vi "Complete Measurament RT (with backnoise remove).vi"() -> ()   [LabVIEW 2014]
uses:
  <vilib>/Platform/TimedLoop/XDataNode/timing_clust.ctl
  <vilib>/Platform/TimedLoop/XDataNode/nitl_modes.ctl
  <vilib>/Platform/TimedLoop/XDataNode/wakeup.ctl
  <vilib>/Analysis/3filter.llb/Filter Passband Type.ctl
  <vilib>/Analysis/Matrix/Datatypes/RealMatrix.ctl
  <vilib>/FPGAPlugInAG/sbRIO-9636/niLvFpga_Open_sbRIO-9636.vi
  <vilib>/rvi/interface/common/dynamic/niFpgaDynamicAddResources.vi
  <vilib>/FPGAPlugInAG/Dynamic/niLvFpga_Reset_Dynamic.vi
  <vilib>/Utility/error.llb/Error Cluster From Error Code.vi
  <vilib>/rvi/errors/niLvFpgaAdjustHostInterfaceError.vi
  <vilib>/Analysis/3filter.llb/Butterworth Filter (DBL).vi
  <vilib>/rvi/interface/common/niFpgaWaitOnOcc.vi
  <vilib>/FPGAPlugInAG/Dynamic/niLvFpga_Run_Dynamic.vi
  <vilib>/FPGAPlugInAG/Dynamic/niLvFpga_Abort_Dynamic.vi
  <vilib>/FPGAPlugInAG/Dynamic/niLvFpga_Close_Dynamic.vi
  <vilib>/rvi/interface/nirviOpenFPGA/nirviOpenFPGA.xnode
  FPGA Bitfiles/LaserDistanceSen_FPGATarget_N-ParametricDoub_hYmJGfBA0FM.lvbitx
  FPGA Target/Test VIs/N-Parametric Double FFT Mesurament Test SLOW (con Sottrazione Fondo).vi
  <vilib>/rvi/interface/nirviMethod/nirviMethod.xnode
  <vilib>/rvi/interface/nirviReadWriteControl/nirviReadWriteControl.xnode
  <vilib>/platform/TimedLoop/XDataNode/XDataNode.xnode
  <vilib>/rvi/interface/nirviCloseFPGA/nirviCloseFPGA.xnode
  <vilib>/FPGAPlugInAG/Dynamic/niLvFpga_ConfigureFifo_Dynamic.vi
  <vilib>/rvi/errors/niLvFpgaMergeErrorWithErrorCode.vi
  <vilib>/FPGAPlugInAG/Dynamic/niLvFpga_StartFifo_Dynamic.vi
  <vilib>/rvi/interface/Simulation/niFpgaSimulationCallBeginRW.vi
  <vilib>/FPGAPlugInAG/Dynamic/niLvFpga_ReadFifo_Dynamic.vi
  <vilib>/Platform/TimedLoop/XDataNode/XDNodeRunTimeDep.lvlib
  NiFpgaLv.dll
  <vilib>/Analysis/NI_AALBase.lvlib
  <vilib>/Analysis/Matrix/NI_Matrix.lvlib
panel:
  out "Array":i32[](array[numeric])
  out "mean distance size":i32
  in  "n-bit (2^nbit medie)":i32=8
  in  "Savitzy golay: polynomial order":i32=3
  in  "Savitzy golay: side points":i32=6
  in  "LowPass Filter: Low cutoff frequency":dbl=1000000.0 format="%#_13g"
  in  "PolyFitting: Poly Grade":dbl=5.0
  in  "SubtractionType":T1(ring)=enum."LowPass"
  out "Fondo Signal":dbl[](graph)
  out "Distance ONLINE":dbl[](graph)
  in  "Low cutoff freq":dbl=200000.0 format="%#_13g"
  in  "Tri Low pass filter":bool
  in  "3 point interpolation algorithm":bool
  in  "Mov mean":bool
  out "moving mean speed":dbl format="%0.7f"
  out "moving standard deviation rel speed":dbl format="%0.7f"
  in  "#movesignal 2":i32=100
  out "moving freq mean":dbl
  in  "Tab Control":enum32{"5 bin", "5 bin mean", "Distance "}(tab)=enum."Distance "
  out "5 bin FALL":T2(graph) caption="5 freq fall"
  out "5 bin RISE":T2(graph)
  out "5 bin mean/std FALL":T3(graph)
  in  "#meanBin":i32=100
  out "5 bin mean/std RISE":T3(graph)
  out "Distance and error":T2(graph)
  out "Speed and error":T2(graph)
  in  "Lin Mes":bool
  in  "step (m)":dbl=0.0001
  out "Max peak-peak error (m)":dbl
  out "Mean error (m)":dbl
  in  "Plot":bool
  in  "Sample /Modulation Frequency":enum32{"40MHz/32KHz", "30MHz/24Khz"}(radio)=enum."30MHz/24Khz"
  in  "#movesignal":i32=100
  out "moving standard deviation rel":dbl format="%0.7f"
  out "moving mean":dbl format="%0.7f"
  out "StdDev Rel 1":dbl
  out "StdDev Rel 2":dbl
  out "Warning":bool
  out "Velocity (m/s)":dbl
  out "Distance (m)":dbl
  out "Mean Frequency":dbl
  out "Rise array size":i32
  out "Fall array size":i32
  out "Mean Frequency Rising (Hz)":dbl
  out "Mean Frequency Falling (Hz)":dbl
  in  "tieni premuto per":i32=100
  in  "Triangular Multiply Factor":dbl[](array[numeric])=[1.0, 0.8, 0.95, 0.85, 0.9]
  out "RISING Second Edge N-FFT":dbl[](graph)
  in  "Enable triangular scaling":bool=TRUE
  in  "Triangolo dritto?":bool
  out "FALLING First Edge N-FFT":dbl[](graph)
  in  "#Signals":u32(slide)=5 scale=1.0..5.0
  in  "stop":bool
  in  "Initial Latency points":u32(slide)=260 scale=0.0..1249.0
  out "Elements Remaining FFT":u32
  out "Elements Remaining Signal":u32
  out "N-Signals":dbl[](graph)
  in  "Snapshot":bool
  in  "Windowing":T4(ring)=enum."Hanning"
  in  "first bin":i32=5
  in  "last bin":i32=255
  in  "lower limit 2":u32(slide)=738 scale=625.0..738.0
  in  "lower limit 1":u32(slide)=113 scale=0.0..113.0
  # "SOTTRAZIONE FONDO"
  # "OFFLINE parameters"
  # "200k/400k"
  # "Max Detection FFT bin range"
  # "WARNING:\nOnce pressed wait untill the end of operation"
  # "Distance"
  # "Mean"
  # "Velocity"
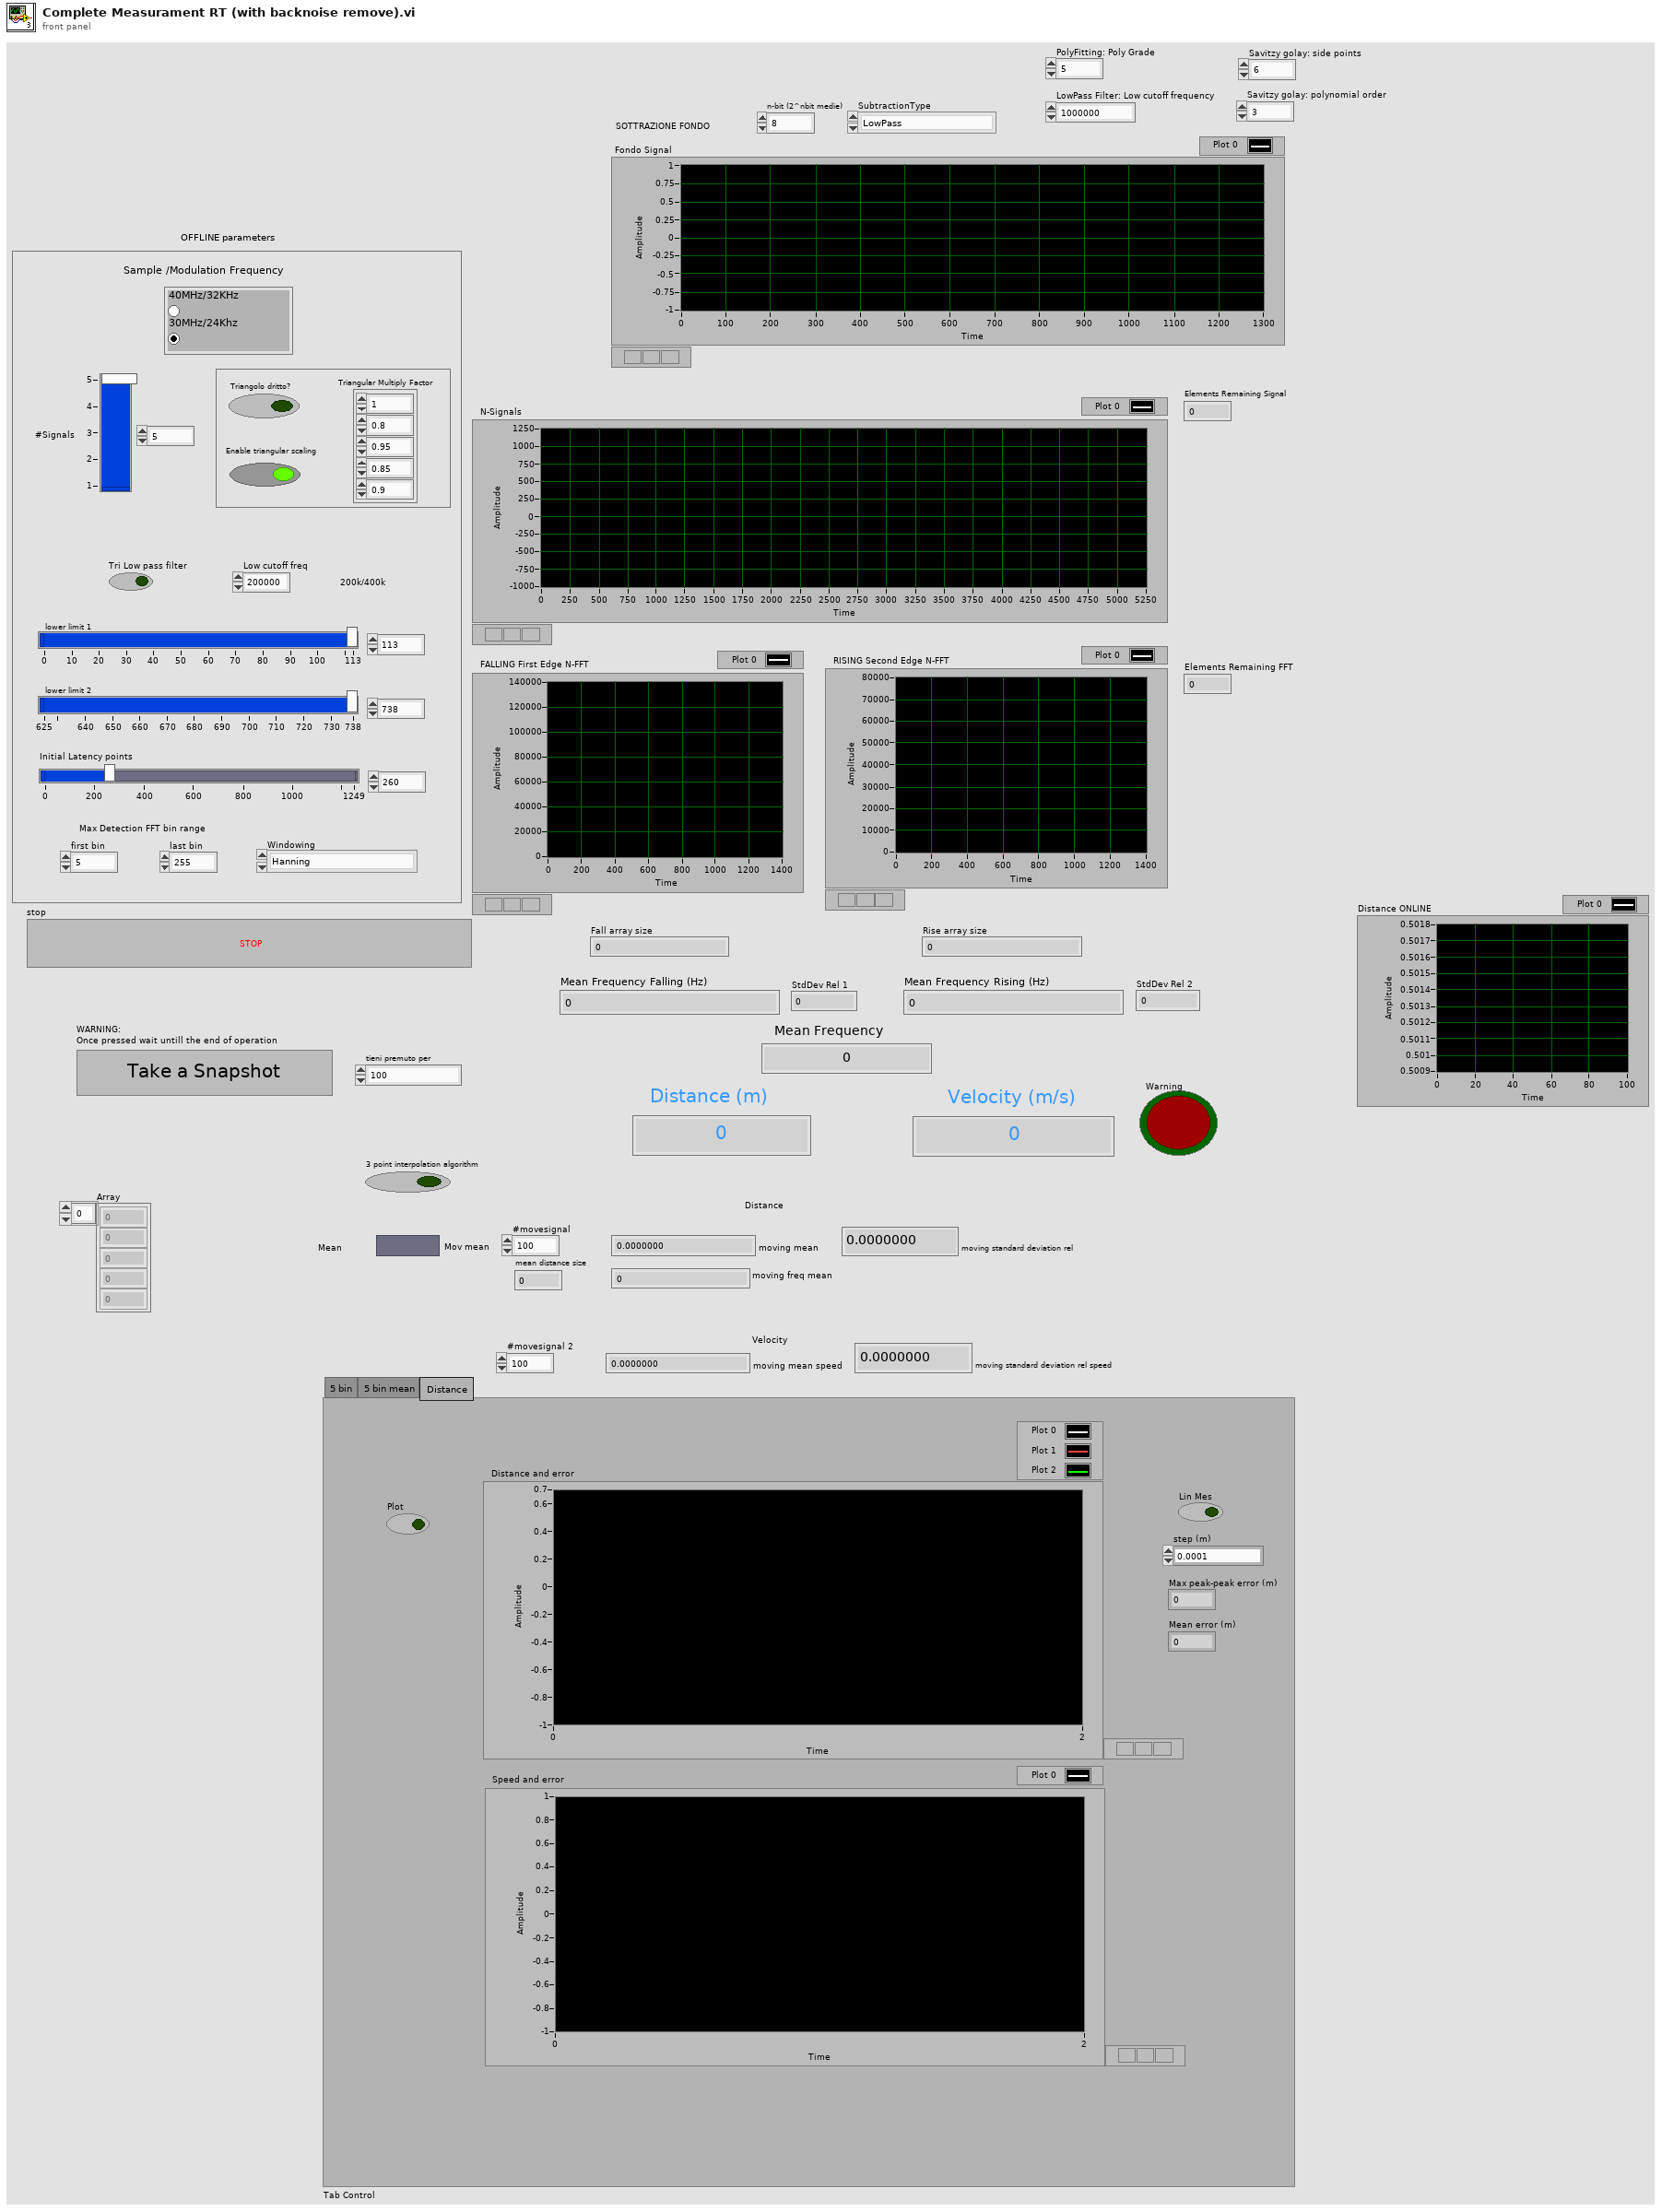
[diagram p1: front panel]
types:
  T1 = enum16{"NoSubtract", "StartingCurve", "LowPass", "PolyFitting", "SavGolay"}
  T2 = cluster{"[0]":dbl, "[1]":dbl, "[2]":dbl, "[3]":dbl, "[4]":dbl, "[5]":dbl, "[6]":dbl, "[7]":dbl, "[8]":dbl}
  T3 = cluster{"Array[0]":dbl, "Array[1]":dbl, "Array[2]":dbl, "Array[3]":dbl, "Array[4]":dbl, "Array[5]":dbl, "Array[6]":dbl, "Array[7]":dbl, "Array[8]":dbl}
  T4 = enum16{"None", "Hanning", "Hamming", "Blackman", "Blackman-Harris"}
  T5 = typedef "NI_AALBase.lvlib/Filter Passband Type.ctl" = enum32{"Lowpass", "Highpass", "Bandpass", "Bandstop"}
  T6 = typedef "XDNodeRunTimeDep.lvlib/timing_clust.ctl" = cluster{"Expected End [f-1]":u64, "Actual End [f-1]":u64, "Finished Late? [f-1]":bool, "Expected End [i-1]":u64, "Actual End [i-1]":u64, "Finished Late? [i-1]":bool, "Expected Start [i]":u64, "Actual Start [i]":u64, "Expected Start [f]":u64, "Actual Start [f]":u64, "Source Name":string, "Structure Name":string, "Period":i64, "Deadline":i64, "Offset":i64, "Start":i64, "Priority":i32, "Timeout":i32, "Mode":T7, "Wakeup Reason":T8, "Error":errorcluster, "Source Type":string, "Secondary Source Type":string, "Global End Time":u64, "Global Start Time":u64, "Frame Duration":u64, "Iteration Duration":u64, "Assigned CPU":i32, "I/O Scan Engine Mode":u32}
  T7 = typedef "XDNodeRunTimeDep.lvlib/nitl_modes.ctl" = enum32{"No Change", "Process missed periods, maintain original phase", "Discard missed periods, maintain original phase", "Process missed periods, ignore original phase", "Discard missed periods, ignore original phase"}
  T8 = typedef "XDNodeRunTimeDep.lvlib/wakeup.ctl" = enum32{"Normal", "Aborted", "Asynchronous wakeup", "Timing source error", "Timed loop error", "Timeout"}
  T9 = typedef "NI_Matrix.lvlib/RealMatrix.ctl" = dbl[][]
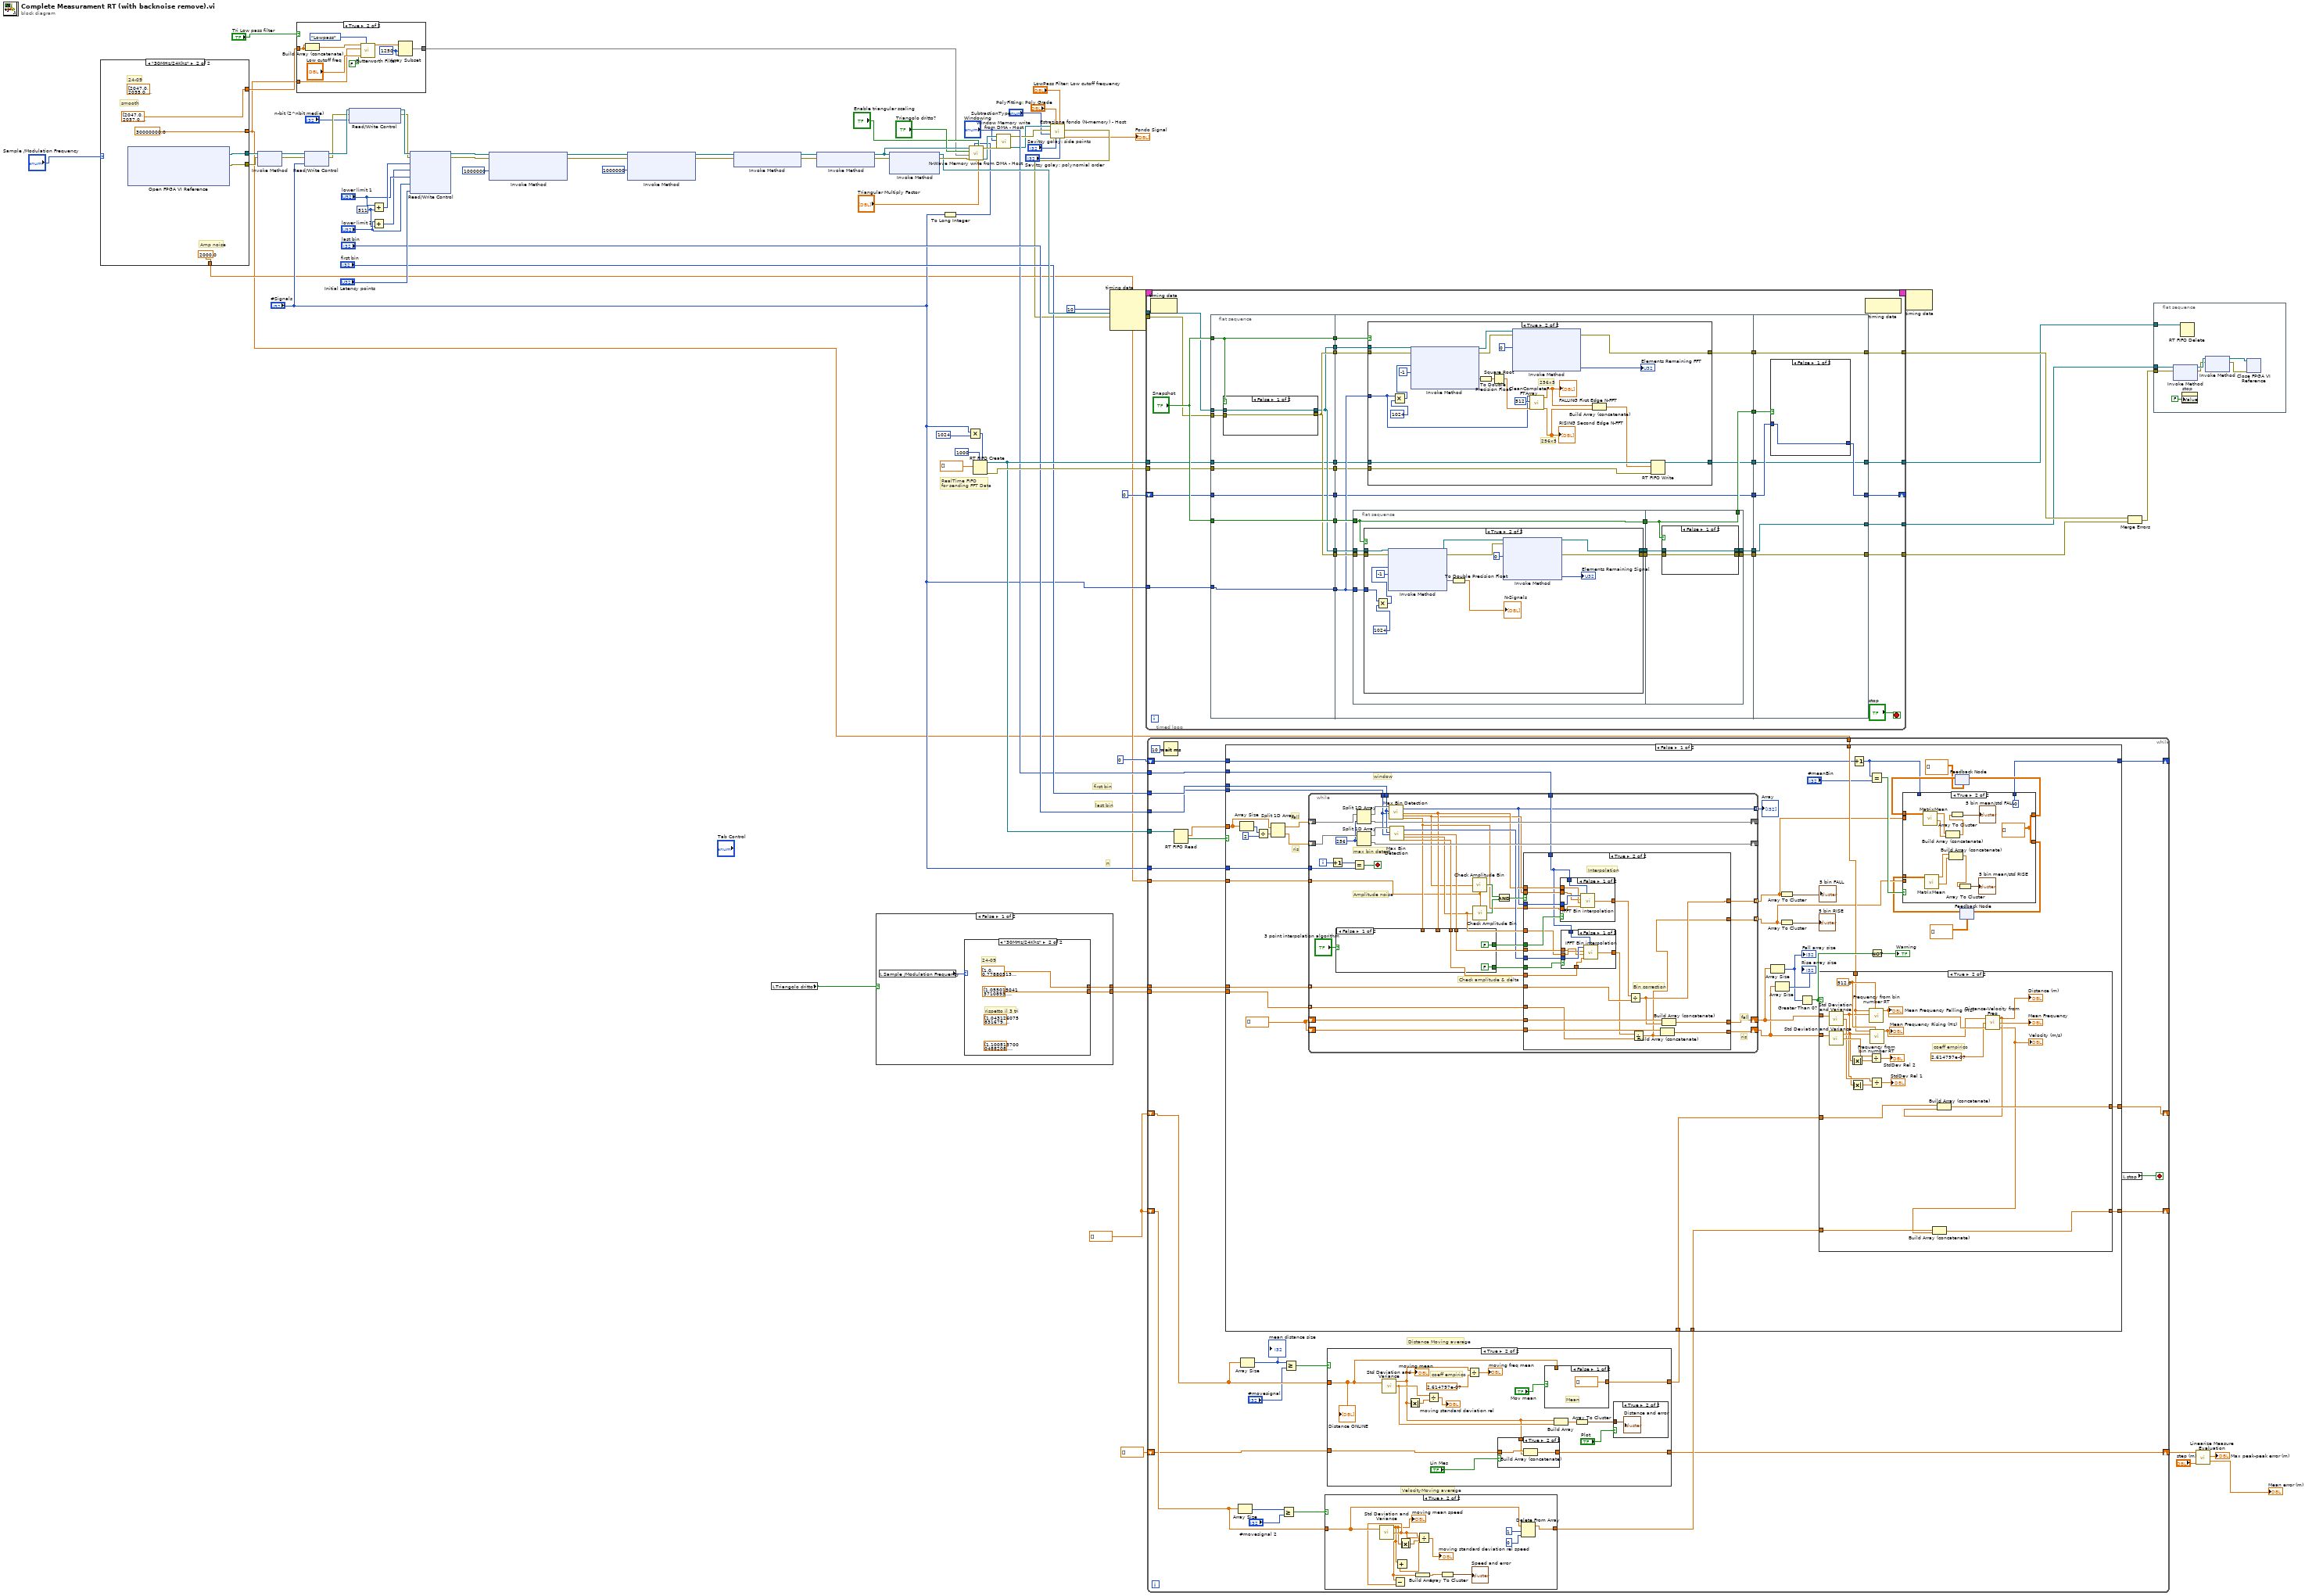
[diagram p0: block diagram]
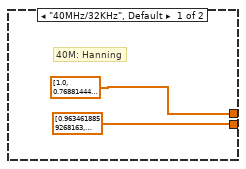
[diagram p3: hidden frame]
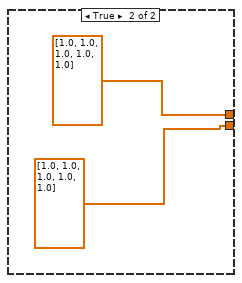
[diagram p4: hidden frame]
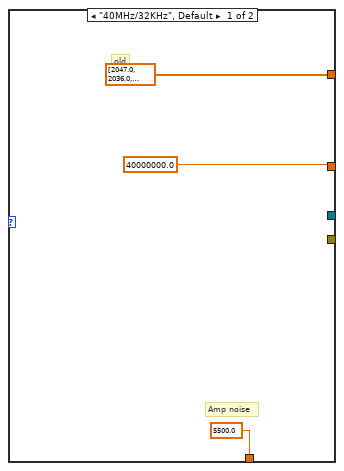
[diagram p5: hidden frame]
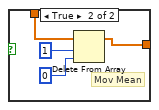
[diagram p10: hidden frame]
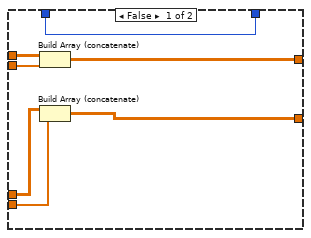
[diagram p11: hidden frame]
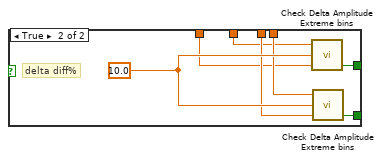
[diagram p13: hidden frame]
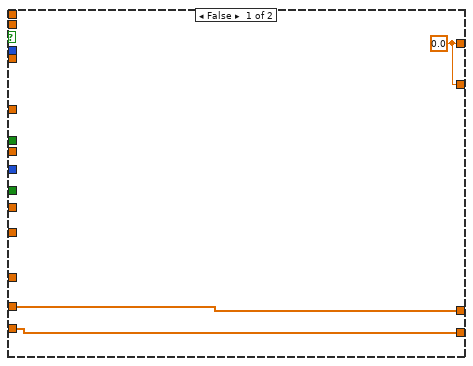
[diagram p14: hidden frame]
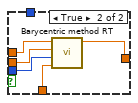
[diagram p15: hidden frame]
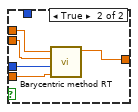
[diagram p16: hidden frame]
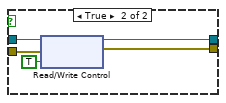
[diagram p18: hidden frame]
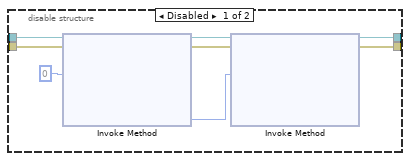
[diagram p20: hidden frame]
diagram:
  w25 = dbl[] [] ("appended array")
  w75 = u32 511 ("y")
  # "n"
  # "last bin"
  # "first bin"
  # "RealTime FIFO \nfor sending FFT Data"
  n1 = case shown="\"30MHz/24Khz\"" "Sample /Modulation Frequency" {
    tunnel: [_ w87] -> w50
    tunnel: [_ w86] -> w49
    tunnel: [40000000.0 30000000.0] -> w21
    tunnel: [5500.0 ("Threshold Amp") 2000.0 ("Threshold Amp")] -> w26
    tunnel: [dbl[] [2047.0, 2036.0, 2024.0, 2013.0, 2002.0, 1990.0, 1979.0, 1968.0, 1956.0, 1945.0, 1934.0, 1923.0, 1912.0, 1900.0, 1889.0, 1878.0, 1867.0, 1856.0, 1845.0, 1833.0, 1822.0, 1811.0, 1800.0, 1789.0, 1778.0, 1767.0, 1756.0, 1745.0, 1734.0, 1723.0, 1712.0, 1702.0, 1691.0, 1680.0, 1669.0, 1658.0, 1647.0, 1636.0, 1626.0, 1615.0, 1604.0, 1593.0, 1583.0, 1572.0, 1561.0, 1550.0, 1540.0, 1529.0, 1518.0, 1508.0, 1497.0, 1487.0, 1476.0, 1465.0, 1455.0, 1444.0, 1434.0, 1423.0, 1413.0, 1402.0, 1392.0, 1381.0, 1371.0, 1360.0, 1350.0, 1340.0, 1329.0, 1319.0, 1309.0, 1298.0, 1288.0, 1278.0, 1267.0, 1257.0, 1247.0, 1237.0, 1226.0, 1216.0, 1206.0, 1196.0, 1186.0, 1176.0, 1165.0, 1155.0, 1145.0, 1135.0, 1125.0, 1115.0, 1105.0, 1095.0, 1085.0, 1075.0, 1065.0, 1055.0, 1045.0, 1035.0, 1025.0, 1015.0, 1006.0, 996.0, 986.0, 976.0, 966.0, 956.0, 947.0, 937.0, 927.0, 917.0, 908.0, 898.0, 888.0, 879.0, 869.0, 859.0, 850.0, 837.0, 826.0, 816.0, 804.0, 796.0, 788.0, 778.0, 769.0, 758.0, 750.0, 743.0, 733.0, 724.0, 717.0, 709.0, 701.0, 693.0, 686.0, 677.0, 669.0, 661.0, 653.0, 645.0, 638.0, 630.0, 622.0, 615.0, 607.0, 599.0, 592.0, 583.0, 576.0, 569.0, 561.0, 554.0, 547.0, 539.0, 532.0, 525.0, 518.0, 509.0, 501.0, 492.0, 486.0, 478.0, 471.0, 463.0, 456.0, 450.0, 442.0, 435.0, 429.0, 421.0, 415.0, 408.0, 401.0, 394.0, 388.0, 381.0, 375.0, 368.0, 361.0, 355.0, 349.0, 342.0, 336.0, 330.0, 323.0, 317.0, 311.0, 304.0, 298.0, 292.0, 286.0, 279.0, 273.0, 267.0, 261.0, 255.0, 249.0, 242.0, 236.0, 230.0, 224.0, 218.0, 212.0, 206.0, 200.0, 194.0, 187.0, 181.0, 175.0, 169.0, 163.0, 157.0, 150.0, 144.0, 138.0, 132.0, 125.0, 119.0, 113.0, 107.0, 101.0, 95.0, 88.0, 82.0, 77.0, 71.0, 65.0, 59.0, 53.0, 47.0, 41.0, 35.0, 29.0, 23.0, 18.0, 11.0, 6.0, 0.0, -6.0, -12.0, -18.0, -23.0, -29.0, -35.0, -41.0, -47.0, -52.0, -58.0, -64.0, -69.0, -75.0, -81.0, -87.0, -92.0, -98.0, -104.0, -109.0, -115.0, -121.0, -126.0, -132.0, -138.0, -144.0, -149.0, -155.0, -161.0, -166.0, -172.0, -177.0, -183.0, -189.0, -194.0, -200.0, -205.0, -211.0, -216.0, -222.0, -227.0, -233.0, -238.0, -244.0, -249.0, -255.0, -260.0, -266.0, -271.0, -277.0, -283.0, -288.0, -294.0, -299.0, -304.0, -310.0, -315.0, -321.0, -326.0, -331.0, -337.0, -342.0, -348.0, -353.0, -358.0, -364.0, -369.0, -375.0, -380.0, -385.0, -391.0, -396.0, -402.0, -407.0, -413.0, -418.0, -423.0, -429.0, -434.0, -439.0, -445.0, -450.0, -456.0, -461.0, -466.0, -472.0, -477.0, -483.0, -488.0, -493.0, -499.0, -504.0, -510.0, -515.0, -520.0, -526.0, -531.0, -537.0, -542.0, -548.0, -553.0, -558.0, -564.0, -569.0, -574.0, -580.0, -585.0, -590.0, -596.0, -601.0, -606.0, -612.0, -617.0, -622.0, -628.0, -633.0, -638.0, -644.0, -649.0, -654.0, -660.0, -665.0, -670.0, -676.0, -681.0, -686.0, -692.0, -697.0, -702.0, -708.0, -713.0, -718.0, -723.0, -729.0, -734.0, -739.0, -744.0, -750.0, -755.0, -760.0, -765.0, -771.0, -776.0, -781.0, -786.0, -792.0, -797.0, -802.0, -807.0, -812.0, -818.0, -823.0, -828.0, -833.0, -839.0, -844.0, -849.0, -854.0, -859.0, -865.0, -870.0, -875.0, -880.0, -885.0, -891.0, -896.0, -901.0, -906.0, -911.0, -916.0, -922.0, -927.0, -932.0, -937.0, -943.0, -948.0, -953.0, -958.0, -963.0, -969.0, -974.0, -979.0, -984.0, -989.0, -995.0, -1000.0, -1005.0, -1010.0, -1015.0, -1021.0, -1026.0, -1031.0, -1036.0, -1041.0, -1047.0, -1052.0, -1057.0, -1062.0, -1067.0, -1073.0, -1078.0, -1083.0, -1088.0, -1093.0, -1099.0, -1104.0, -1109.0, -1114.0, -1119.0, -1124.0, -1130.0, -1135.0, -1140.0, -1145.0, -1150.0, -1156.0, -1161.0, -1166.0, -1171.0, -1176.0, -1182.0, -1187.0, -1192.0, -1197.0, -1202.0, -1207.0, -1213.0, -1218.0, -1223.0, -1228.0, -1233.0, -1238.0, -1244.0, -1249.0, -1254.0, -1259.0, -1264.0, -1269.0, -1275.0, -1280.0, -1285.0, -1290.0, -1295.0, -1300.0, -1305.0, -1311.0, -1316.0, -1321.0, -1326.0, -1331.0, -1336.0, -1342.0, -1347.0, -1352.0, -1357.0, -1362.0, -1367.0, -1372.0, -1378.0, -1383.0, -1388.0, -1393.0, -1398.0, -1403.0, -1408.0, -1414.0, -1419.0, -1424.0, -1429.0, -1434.0, -1439.0, -1444.0, -1450.0, -1455.0, -1460.0, -1465.0, -1470.0, -1475.0, -1480.0, -1486.0, -1491.0, -1496.0, -1501.0, -1506.0, -1511.0, -1516.0, -1522.0, -1527.0, -1532.0, -1537.0, -1542.0, -1547.0, -1552.0, -1558.0, -1563.0, -1568.0, -1573.0, -1578.0, -1583.0, -1588.0, -1593.0, -1599.0, -1604.0, -1609.0, -1614.0, -1619.0, -1624.0, -1629.0, -1634.0, -1640.0, -1645.0, -1650.0, -1655.0, -1660.0, -1665.0, -1670.0, -1675.0, -1681.0, -1686.0, -1691.0, -1696.0, -1701.0, -1706.0, -1711.0, -1716.0, -1722.0, -1727.0, -1732.0, -1737.0, -1742.0, -1747.0, -1752.0, -1757.0, -1762.0, -1768.0, -1773.0, -1778.0, -1783.0, -1788.0, -1793.0, -1798.0, -1803.0, -1808.0, -1814.0, -1819.0, -1824.0, -1829.0, -1834.0, -1839.0, -1844.0, -1849.0, -1854.0, -1859.0, -1865.0, -1870.0, -1875.0, -1880.0, -1885.0, -1890.0, -1895.0, -1900.0, -1905.0, -1911.0, -1916.0, -1921.0, -1926.0, -1931.0, -1936.0, -1941.0, -1946.0, -1951.0, -1956.0, -1961.0, -1967.0, -1972.0, -1977.0, -1982.0, -1987.0, -1992.0, -1997.0, -2002.0, -2007.0, -2012.0, -2017.0, -2023.0, -2028.0, -2033.0, -2038.0, -2043.0, -2048.0, -2047.0, -2034.0, -2021.0, -2009.0, -1996.0, -1983.0, -1970.0, -1957.0, -1945.0, -1932.0, -1919.0, -1907.0, -1894.0, -1881.0, -1869.0, -1856.0, -1844.0, -1831.0, -1819.0, -1806.0, -1794.0, -1781.0, -1769.0, -1757.0, -1744.0, -1732.0, -1719.0, -1707.0, -1695.0, -1682.0, -1670.0, -1658.0, -1646.0, -1634.0, -1621.0, -1609.0, -1597.0, -1585.0, -1573.0, -1561.0, -1549.0, -1537.0, -1525.0, -1513.0, -1501.0, -1489.0, -1477.0, -1465.0, -1453.0, -1441.0, -1429.0, -1417.0, -1405.0, -1394.0, -1382.0, -1370.0, -1358.0, -1347.0, -1335.0, -1323.0, -1312.0, -1300.0, -1288.0, -1277.0, -1265.0, -1254.0, -1242.0, -1231.0, -1219.0, -1208.0, -1196.0, -1185.0, -1173.0, -1162.0, -1150.0, -1139.0, -1128.0, -1116.0, -1105.0, -1094.0, -1083.0, -1071.0, -1060.0, -1049.0, -1038.0, -1027.0, -1015.0, -1004.0, -993.0, -982.0, -971.0, -960.0, -949.0, -938.0, -927.0, -916.0, -905.0, -894.0, -883.0, -873.0, -862.0, -851.0, -840.0, -829.0, -819.0, -808.0, -797.0, -786.0, -776.0, -765.0, -754.0, -744.0, -733.0, -722.0, -712.0, -697.0, -685.0, -674.0, -661.0, -652.0, -643.0, -632.0, -622.0, -610.0, -602.0, -594.0, -583.0, -574.0, -566.0, -558.0, -550.0, -542.0, -534.0, -525.0, -516.0, -507.0, -499.0, -491.0, -483.0, -475.0, -467.0, -459.0, -451.0, -443.0, -435.0, -426.0, -419.0, -411.0, -404.0, -396.0, -388.0, -381.0, -373.0, -366.0, -359.0, -349.0, -341.0, -331.0, -325.0, -317.0, -309.0, -301.0, -295.0, -288.0, -280.0, -273.0, -266.0, -259.0, -252.0, -246.0, -239.0, -231.0, -225.0, -219.0, -212.0, -205.0, -199.0, -192.0, -186.0, -180.0, -173.0, -167.0, -161.0, -155.0, -148.0, -142.0, -136.0, -130.0, -124.0, -118.0, -112.0, -106.0, -100.0, -94.0, -88.0, -82.0, -76.0, -70.0, -64.0, -58.0, -52.0, -46.0, -40.0, -34.0, -28.0, -21.0, -15.0, -9.0, -3.0, 2.0, 9.0, 15.0, 21.0, 27.0, 33.0, 39.0, 45.0, 51.0, 57.0, 63.0, 69.0, 75.0, 81.0, 86.0, 92.0, 98.0, 103.0, 110.0, 116.0, 121.0, 127.0, 133.0, 138.0, 144.0, 149.0, 155.0, 161.0, 166.0, 172.0, 177.0, 183.0, 189.0, 194.0, 200.0, 205.0, 211.0, 216.0, 221.0, 227.0, 232.0, 238.0, 243.0, 249.0, 254.0, 259.0, 265.0, 270.0, 276.0, 281.0, 286.0, 292.0, 297.0, 303.0, 308.0, 314.0, 319.0, 324.0, 329.0, 335.0, 340.0, 345.0, 351.0, 356.0, 361.0, 366.0, 371.0, 377.0, 382.0, 387.0, 392.0, 397.0, 403.0, 408.0, 413.0, 418.0, 423.0, 429.0, 434.0, 439.0, 444.0, 449.0, 454.0, 459.0, 464.0, 469.0, 474.0, 479.0, 484.0, 489.0, 494.0, 499.0, 504.0, 509.0, 514.0, 520.0, 525.0, 530.0, 535.0, 540.0, 545.0, 550.0, 555.0, 560.0, 565.0, 570.0, 575.0, 580.0, 585.0, 590.0, 595.0, 600.0, 605.0, 610.0, 615.0, 620.0, 625.0, 630.0, 636.0, 641.0, 646.0, 651.0, 656.0, 661.0, 666.0, 671.0, 676.0, 681.0, 686.0, 691.0, 696.0, 701.0, 706.0, 711.0, 716.0, 721.0, 726.0, 731.0, 736.0, 741.0, 746.0, 751.0, 756.0, 761.0, 765.0, 770.0, 775.0, 780.0, 785.0, 790.0, 795.0, 800.0, 805.0, 810.0, 815.0, 820.0, 825.0, 829.0, 834.0, 839.0, 844.0, 849.0, 854.0, 859.0, 864.0, 868.0, 873.0, 878.0, 883.0, 888.0, 893.0, 897.0, 902.0, 907.0, 912.0, 917.0, 921.0, 926.0, 931.0, 936.0, 941.0, 945.0, 950.0, 955.0, 960.0, 965.0, 969.0, 974.0, 979.0, 984.0, 988.0, 993.0, 998.0, 1003.0, 1007.0, 1012.0, 1017.0, 1022.0, 1027.0, 1031.0, 1036.0, 1041.0, 1046.0, 1051.0, 1055.0, 1060.0, 1065.0, 1070.0, 1075.0, 1079.0, 1084.0, 1089.0, 1094.0, 1098.0, 1103.0, 1108.0, 1113.0, 1118.0, 1122.0, 1127.0, 1132.0, 1137.0, 1141.0, 1146.0, 1151.0, 1156.0, 1161.0, 1165.0, 1170.0, 1175.0, 1180.0, 1184.0, 1189.0, 1194.0, 1199.0, 1204.0, 1208.0, 1213.0, 1218.0, 1223.0, 1227.0, 1232.0, 1237.0, 1242.0, 1246.0, 1251.0, 1256.0, 1261.0, 1265.0, 1270.0, 1275.0, 1280.0, 1284.0, 1289.0, 1294.0, 1299.0, 1303.0, 1308.0, 1313.0, 1318.0, 1322.0, 1327.0, 1332.0, 1336.0, 1341.0, 1346.0, 1351.0, 1355.0, 1360.0, 1365.0, 1370.0, 1374.0, 1379.0, 1384.0, 1388.0, 1393.0, 1398.0, 1403.0, 1407.0, 1412.0, 1417.0, 1421.0, 1426.0, 1431.0, 1436.0, 1440.0, 1445.0, 1450.0, 1454.0, 1459.0, 1464.0, 1469.0, 1473.0, 1478.0, 1483.0, 1487.0, 1492.0, 1497.0, 1502.0, 1506.0, 1511.0, 1516.0, 1520.0, 1525.0, 1530.0, 1535.0, 1539.0, 1544.0, 1549.0, 1553.0, 1558.0, 1563.0, 1567.0, 1572.0, 1577.0, 1582.0, 1586.0, 1591.0, 1596.0, 1600.0, 1605.0, 1610.0, 1614.0, 1619.0, 1624.0, 1628.0, 1633.0, 1638.0, 1643.0, 1647.0, 1652.0, 1657.0, 1661.0, 1666.0, 1671.0, 1675.0, 1680.0, 1685.0, 1689.0, 1694.0, 1699.0, 1703.0, 1708.0, 1713.0, 1717.0, 1722.0, 1727.0, 1731.0, 1736.0, 1741.0, 1746.0, 1750.0, 1755.0, 1760.0, 1764.0, 1769.0, 1774.0, 1778.0, 1783.0, 1788.0, 1792.0, 1797.0, 1802.0, 1806.0, 1811.0, 1816.0, 1820.0, 1825.0, 1830.0, 1834.0, 1839.0, 1844.0, 1848.0, 1853.0, 1858.0, 1862.0, 1867.0, 1871.0, 1876.0, 1881.0, 1885.0, 1890.0, 1895.0, 1899.0, 1904.0, 1909.0, 1913.0, 1918.0, 1923.0, 1927.0, 1932.0, 1937.0, 1941.0, 1946.0, 1951.0, 1955.0, 1960.0, 1965.0, 1969.0, 1974.0, 1978.0, 1983.0, 1988.0, 1992.0, 1997.0, 2002.0, 2006.0, 2011.0, 2016.0, 2020.0, 2025.0, 2029.0, 2034.0, 2039.0, 2043.0, 2048.0] ("Complete SkewTri") dbl[] [2047.0, 2037.0, 2027.0, 2018.0, 2008.0, 1998.0, 1989.0, 1979.0, 1969.0, 1960.0, 1950.0, 1940.0, 1931.0, 1921.0, 1911.0, 1902.0, 1892.0, 1882.0, 1873.0, 1863.0, 1854.0, 1844.0, 1835.0, 1825.0, 1816.0, 1806.0, 1797.0, 1787.0, 1778.0, 1768.0, 1759.0, 1749.0, 1740.0, 1730.0, 1721.0, 1711.0, 1702.0, 1693.0, 1683.0, 1674.0, 1665.0, 1655.0, 1646.0, 1637.0, 1627.0, 1618.0, 1609.0, 1599.0, 1590.0, 1581.0, 1572.0, 1562.0, 1553.0, 1544.0, 1535.0, 1525.0, 1516.0, 1507.0, 1498.0, 1489.0, 1479.0, 1470.0, 1461.0, 1452.0, 1443.0, 1434.0, 1425.0, 1416.0, 1407.0, 1398.0, 1388.0, 1379.0, 1370.0, 1361.0, 1352.0, 1343.0, 1334.0, 1325.0, 1316.0, 1307.0, 1299.0, 1290.0, 1281.0, 1272.0, 1263.0, 1254.0, 1245.0, 1236.0, 1227.0, 1218.0, 1210.0, 1201.0, 1192.0, 1183.0, 1174.0, 1166.0, 1157.0, 1148.0, 1139.0, 1130.0, 1122.0, 1113.0, 1104.0, 1096.0, 1087.0, 1078.0, 1069.0, 1061.0, 1052.0, 1043.0, 1035.0, 1026.0, 1018.0, 1009.0, 1000.0, 992.0, 983.0, 975.0, 966.0, 958.0, 950.0, 941.0, 933.0, 925.0, 917.0, 908.0, 900.0, 892.0, 884.0, 876.0, 868.0, 860.0, 852.0, 844.0, 837.0, 829.0, 821.0, 813.0, 805.0, 798.0, 790.0, 782.0, 775.0, 767.0, 760.0, 752.0, 745.0, 737.0, 730.0, 722.0, 715.0, 707.0, 700.0, 693.0, 685.0, 678.0, 671.0, 664.0, 656.0, 649.0, 642.0, 635.0, 628.0, 621.0, 613.0, 606.0, 599.0, 592.0, 585.0, 578.0, 571.0, 564.0, 557.0, 550.0, 543.0, 537.0, 530.0, 523.0, 516.0, 509.0, 502.0, 495.0, 489.0, 482.0, 475.0, 468.0, 462.0, 455.0, 448.0, 442.0, 435.0, 428.0, 422.0, 415.0, 408.0, 402.0, 395.0, 389.0, 382.0, 375.0, 369.0, 362.0, 356.0, 349.0, 343.0, 336.0, 330.0, 324.0, 317.0, 311.0, 304.0, 298.0, 291.0, 285.0, 279.0, 272.0, 266.0, 260.0, 253.0, 247.0, 241.0, 234.0, 228.0, 222.0, 215.0, 209.0, 203.0, 197.0, 190.0, 184.0, 178.0, 172.0, 165.0, 159.0, 153.0, 147.0, 141.0, 135.0, 128.0, 122.0, 116.0, 110.0, 104.0, 98.0, 92.0, 85.0, 79.0, 73.0, 67.0, 61.0, 55.0, 49.0, 43.0, 37.0, 31.0, 25.0, 19.0, 13.0, 7.0, 1.0, -5.0, -11.0, -17.0, -23.0, -29.0, -35.0, -41.0, -47.0, -53.0, -59.0, -65.0, -71.0, -77.0, -83.0, -89.0, -95.0, -101.0, -107.0, -113.0, -119.0, -124.0, -130.0, -136.0, -142.0, -148.0, -154.0, -160.0, -166.0, -172.0, -177.0, -183.0, -189.0, -195.0, -201.0, -207.0, -212.0, -218.0, -224.0, -230.0, -236.0, -242.0, -247.0, -253.0, -259.0, -265.0, -271.0, -276.0, -282.0, -288.0, -294.0, -300.0, -305.0, -311.0, -317.0, -323.0, -328.0, -334.0, -340.0, -346.0, -351.0, -357.0, -363.0, -369.0, -374.0, -380.0, -386.0, -392.0, -397.0, -403.0, -409.0, -414.0, -420.0, -426.0, -432.0, -437.0, -443.0, -449.0, -454.0, -460.0, -466.0, -471.0, -477.0, -483.0, -489.0, -494.0, -500.0, -506.0, -511.0, -517.0, -523.0, -528.0, -534.0, -540.0, -545.0, -551.0, -557.0, -562.0, -568.0, -573.0, -579.0, -585.0, -590.0, -596.0, -602.0, -607.0, -613.0, -619.0, -624.0, -630.0, -635.0, -641.0, -647.0, -652.0, -658.0, -664.0, -669.0, -675.0, -680.0, -686.0, -692.0, -697.0, -703.0, -708.0, -714.0, -720.0, -725.0, -731.0, -737.0, -742.0, -748.0, -753.0, -759.0, -764.0, -770.0, -776.0, -781.0, -787.0, -792.0, -798.0, -804.0, -809.0, -815.0, -820.0, -826.0, -831.0, -837.0, -843.0, -848.0, -854.0, -859.0, -865.0, -871.0, -876.0, -882.0, -887.0, -893.0, -898.0, -904.0, -909.0, -915.0, -921.0, -926.0, -932.0, -937.0, -943.0, -948.0, -954.0, -960.0, -965.0, -971.0, -976.0, -982.0, -987.0, -993.0, -998.0, -1004.0, -1009.0, -1015.0, -1021.0, -1026.0, -1032.0, -1037.0, -1043.0, -1048.0, -1054.0, -1059.0, -1065.0, -1070.0, -1076.0, -1082.0, -1087.0, -1093.0, -1098.0, -1104.0, -1109.0, -1115.0, -1120.0, -1126.0, -1131.0, -1137.0, -1142.0, -1148.0, -1154.0, -1159.0, -1165.0, -1170.0, -1176.0, -1181.0, -1187.0, -1192.0, -1198.0, -1203.0, -1209.0, -1214.0, -1220.0, -1225.0, -1231.0, -1237.0, -1242.0, -1248.0, -1253.0, -1259.0, -1264.0, -1270.0, -1275.0, -1281.0, -1286.0, -1292.0, -1297.0, -1303.0, -1308.0, -1314.0, -1319.0, -1325.0, -1331.0, -1336.0, -1342.0, -1347.0, -1353.0, -1358.0, -1364.0, -1369.0, -1375.0, -1380.0, -1386.0, -1391.0, -1397.0, -1402.0, -1408.0, -1413.0, -1419.0, -1424.0, -1430.0, -1435.0, -1441.0, -1447.0, -1452.0, -1458.0, -1463.0, -1469.0, -1474.0, -1480.0, -1485.0, -1491.0, -1496.0, -1502.0, -1507.0, -1513.0, -1518.0, -1524.0, -1529.0, -1535.0, -1540.0, -1546.0, -1551.0, -1557.0, -1563.0, -1568.0, -1574.0, -1579.0, -1585.0, -1590.0, -1596.0, -1601.0, -1607.0, -1612.0, -1618.0, -1623.0, -1629.0, -1634.0, -1640.0, -1645.0, -1651.0, -1656.0, -1662.0, -1667.0, -1673.0, -1678.0, -1684.0, -1689.0, -1695.0, -1701.0, -1706.0, -1712.0, -1717.0, -1723.0, -1728.0, -1734.0, -1739.0, -1745.0, -1750.0, -1756.0, -1761.0, -1767.0, -1772.0, -1778.0, -1783.0, -1789.0, -1794.0, -1800.0, -1805.0, -1811.0, -1816.0, -1822.0, -1827.0, -1833.0, -1838.0, -1844.0, -1849.0, -1855.0, -1861.0, -1866.0, -1872.0, -1877.0, -1883.0, -1888.0, -1894.0, -1899.0, -1905.0, -1910.0, -1916.0, -1921.0, -1927.0, -1932.0, -1938.0, -1943.0, -1949.0, -1954.0, -1960.0, -1965.0, -1971.0, -1976.0, -1982.0, -1987.0, -1993.0, -1998.0, -2004.0, -2009.0, -2015.0, -2020.0, -2026.0, -2031.0, -2037.0, -2042.0, -2048.0, -2047.0, -2035.0, -2024.0, -2012.0, -2001.0, -1989.0, -1977.0, -1966.0, -1954.0, -1943.0, -1931.0, -1920.0, -1908.0, -1897.0, -1886.0, -1874.0, -1863.0, -1851.0, -1840.0, -1829.0, -1817.0, -1806.0, -1795.0, -1783.0, -1772.0, -1761.0, -1750.0, -1738.0, -1727.0, -1716.0, -1705.0, -1694.0, -1683.0, -1671.0, -1660.0, -1649.0, -1638.0, -1627.0, -1616.0, -1605.0, -1594.0, -1583.0, -1572.0, -1561.0, -1550.0, -1539.0, -1528.0, -1517.0, -1507.0, -1496.0, -1485.0, -1474.0, -1463.0, -1452.0, -1442.0, -1431.0, -1420.0, -1409.0, -1399.0, -1388.0, -1377.0, -1367.0, -1356.0, -1345.0, -1335.0, -1324.0, -1314.0, -1303.0, -1293.0, -1282.0, -1271.0, -1261.0, -1250.0, -1240.0, -1230.0, -1219.0, -1209.0, -1198.0, -1188.0, -1178.0, -1167.0, -1157.0, -1147.0, -1136.0, -1126.0, -1116.0, -1105.0, -1095.0, -1085.0, -1075.0, -1065.0, -1054.0, -1044.0, -1034.0, -1024.0, -1014.0, -1004.0, -994.0, -984.0, -974.0, -964.0, -954.0, -944.0, -934.0, -924.0, -914.0, -904.0, -894.0, -884.0, -874.0, -864.0, -854.0, -844.0, -835.0, -825.0, -815.0, -806.0, -796.0, -786.0, -777.0, -768.0, -758.0, -749.0, -740.0, -731.0, -722.0, -713.0, -704.0, -695.0, -686.0, -678.0, -669.0, -660.0, -652.0, -643.0, -635.0, -626.0, -618.0, -610.0, -601.0, -593.0, -585.0, -577.0, -569.0, -561.0, -553.0, -545.0, -537.0, -529.0, -521.0, -513.0, -506.0, -498.0, -490.0, -483.0, -475.0, -467.0, -460.0, -452.0, -445.0, -437.0, -430.0, -423.0, -415.0, -408.0, -401.0, -393.0, -386.0, -379.0, -372.0, -365.0, -358.0, -351.0, -343.0, -336.0, -329.0, -322.0, -316.0, -309.0, -302.0, -295.0, -288.0, -281.0, -274.0, -268.0, -261.0, -254.0, -247.0, -241.0, -234.0, -227.0, -221.0, -214.0, -207.0, -201.0, -194.0, -188.0, -181.0, -175.0, -168.0, -162.0, -155.0, -149.0, -143.0, -136.0, -130.0, -123.0, -117.0, -111.0, -104.0, -98.0, -92.0, -86.0, -79.0, -73.0, -67.0, -61.0, -54.0, -48.0, -42.0, -36.0, -30.0, -24.0, -18.0, -11.0, -5.0, 1.0, 7.0, 13.0, 19.0, 25.0, 31.0, 37.0, 43.0, 49.0, 55.0, 61.0, 67.0, 73.0, 78.0, 84.0, 90.0, 96.0, 102.0, 108.0, 114.0, 120.0, 125.0, 131.0, 137.0, 143.0, 149.0, 154.0, 160.0, 166.0, 172.0, 178.0, 183.0, 189.0, 195.0, 200.0, 206.0, 212.0, 218.0, 223.0, 229.0, 235.0, 240.0, 246.0, 251.0, 257.0, 263.0, 268.0, 274.0, 280.0, 285.0, 291.0, 296.0, 302.0, 307.0, 313.0, 319.0, 324.0, 330.0, 335.0, 341.0, 346.0, 352.0, 357.0, 363.0, 368.0, 374.0, 379.0, 385.0, 390.0, 396.0, 401.0, 407.0, 412.0, 418.0, 423.0, 428.0, 434.0, 439.0, 445.0, 450.0, 455.0, 461.0, 466.0, 472.0, 477.0, 482.0, 488.0, 493.0, 499.0, 504.0, 509.0, 515.0, 520.0, 525.0, 531.0, 536.0, 541.0, 547.0, 552.0, 557.0, 563.0, 568.0, 573.0, 579.0, 584.0, 589.0, 594.0, 600.0, 605.0, 610.0, 616.0, 621.0, 626.0, 631.0, 637.0, 642.0, 647.0, 652.0, 658.0, 663.0, 668.0, 673.0, 678.0, 684.0, 689.0, 694.0, 699.0, 705.0, 710.0, 715.0, 720.0, 725.0, 731.0, 736.0, 741.0, 746.0, 751.0, 757.0, 762.0, 767.0, 772.0, 777.0, 782.0, 788.0, 793.0, 798.0, 803.0, 808.0, 813.0, 818.0, 824.0, 829.0, 834.0, 839.0, 844.0, 849.0, 854.0, 860.0, 865.0, 870.0, 875.0, 880.0, 885.0, 890.0, 895.0, 900.0, 906.0, 911.0, 916.0, 921.0, 926.0, 931.0, 936.0, 941.0, 946.0, 951.0, 956.0, 961.0, 967.0, 972.0, 977.0, 982.0, 987.0, 992.0, 997.0, 1002.0, 1007.0, 1012.0, 1017.0, 1022.0, 1027.0, 1032.0, 1037.0, 1042.0, 1047.0, 1052.0, 1058.0, 1063.0, 1068.0, 1073.0, 1078.0, 1083.0, 1088.0, 1093.0, 1098.0, 1103.0, 1108.0, 1113.0, 1118.0, 1123.0, 1128.0, 1133.0, 1138.0, 1143.0, 1148.0, 1153.0, 1158.0, 1163.0, 1168.0, 1173.0, 1178.0, 1183.0, 1188.0, 1193.0, 1198.0, 1203.0, 1208.0, 1213.0, 1218.0, 1223.0, 1228.0, 1233.0, 1238.0, 1243.0, 1248.0, 1253.0, 1258.0, 1263.0, 1268.0, 1273.0, 1278.0, 1283.0, 1287.0, 1292.0, 1297.0, 1302.0, 1307.0, 1312.0, 1317.0, 1322.0, 1327.0, 1332.0, 1337.0, 1342.0, 1347.0, 1352.0, 1357.0, 1362.0, 1367.0, 1372.0, 1377.0, 1382.0, 1387.0, 1391.0, 1396.0, 1401.0, 1406.0, 1411.0, 1416.0, 1421.0, 1426.0, 1431.0, 1436.0, 1441.0, 1446.0, 1451.0, 1456.0, 1460.0, 1465.0, 1470.0, 1475.0, 1480.0, 1485.0, 1490.0, 1495.0, 1500.0, 1505.0, 1510.0, 1515.0, 1519.0, 1524.0, 1529.0, 1534.0, 1539.0, 1544.0, 1549.0, 1554.0, 1559.0, 1564.0, 1568.0, 1573.0, 1578.0, 1583.0, 1588.0, 1593.0, 1598.0, 1603.0, 1608.0, 1612.0, 1617.0, 1622.0, 1627.0, 1632.0, 1637.0, 1642.0, 1647.0, 1652.0, 1656.0, 1661.0, 1666.0, 1671.0, 1676.0, 1681.0, 1686.0, 1691.0, 1695.0, 1700.0, 1705.0, 1710.0, 1715.0, 1720.0, 1725.0, 1729.0, 1734.0, 1739.0, 1744.0, 1749.0, 1754.0, 1759.0, 1763.0, 1768.0, 1773.0, 1778.0, 1783.0, 1788.0, 1793.0, 1797.0, 1802.0, 1807.0, 1812.0, 1817.0, 1822.0, 1826.0, 1831.0, 1836.0, 1841.0, 1846.0, 1851.0, 1856.0, 1860.0, 1865.0, 1870.0, 1875.0, 1880.0, 1884.0, 1889.0, 1894.0, 1899.0, 1904.0, 1909.0, 1913.0, 1918.0, 1923.0, 1928.0, 1933.0, 1938.0, 1942.0, 1947.0, 1952.0, 1957.0, 1962.0, 1966.0, 1971.0, 1976.0, 1981.0, 1986.0, 1990.0, 1995.0, 2000.0, 2005.0, 2010.0, 2014.0, 2019.0, 2024.0, 2029.0, 2034.0, 2038.0, 2043.0, 2048.0] ("Complete SkewTri")] -> w23
    frame "40MHz/32KHz", Default {
      # "old"
      # "Amp noise"
    }
    frame "30MHz/24Khz" {
      (unwired) dbl[] [2047.0, 2035.0, 2022.0, 2010.0, 1997.0, 1985.0, 1972.0, 1960.0, 1948.0, 1935.0, 1923.0, 1911.0, 1899.0, 1886.0, 1874.0, 1862.0, 1850.0, 1838.0, 1825.0, 1813.0, 1801.0, 1789.0, 1777.0, 1765.0, 1753.0, 1741.0, 1729.0, 1717.0, 1705.0, 1693.0, 1681.0, 1669.0, 1657.0, 1645.0, 1634.0, 1622.0, 1610.0, 1598.0, 1586.0, 1575.0, 1563.0, 1551.0, 1540.0, 1528.0, 1516.0, 1505.0, 1493.0, 1481.0, 1470.0, 1458.0, 1447.0, 1435.0, 1424.0, 1412.0, 1401.0, 1389.0, 1378.0, 1366.0, 1355.0, 1344.0, 1332.0, 1321.0, 1310.0, 1298.0, 1287.0, 1276.0, 1265.0, 1253.0, 1242.0, 1231.0, 1220.0, 1209.0, 1198.0, 1186.0, 1175.0, 1164.0, 1153.0, 1142.0, 1131.0, 1120.0, 1109.0, 1098.0, 1087.0, 1076.0, 1065.0, 1055.0, 1044.0, 1033.0, 1022.0, 1011.0, 1000.0, 990.0, 979.0, 968.0, 958.0, 947.0, 936.0, 926.0, 915.0, 904.0, 894.0, 883.0, 873.0, 862.0, 852.0, 841.0, 831.0, 820.0, 810.0, 799.0, 789.0, 778.0, 768.0, 758.0, 747.0, 738.0, 727.0, 719.0, 712.0, 706.0, 700.0, 693.0, 687.0, 680.0, 674.0, 668.0, 661.0, 655.0, 648.0, 642.0, 636.0, 629.0, 623.0, 617.0, 610.0, 604.0, 598.0, 591.0, 584.0, 577.0, 569.0, 560.0, 552.0, 545.0, 538.0, 531.0, 525.0, 519.0, 512.0, 506.0, 500.0, 494.0, 488.0, 482.0, 476.0, 470.0, 464.0, 458.0, 452.0, 446.0, 436.0, 430.0, 424.0, 418.0, 412.0, 406.0, 400.0, 394.0, 388.0, 382.0, 376.0, 370.0, 364.0, 358.0, 352.0, 346.0, 338.0, 332.0, 325.0, 319.0, 313.0, 307.0, 301.0, 295.0, 290.0, 284.0, 278.0, 272.0, 267.0, 261.0, 255.0, 249.0, 244.0, 238.0, 232.0, 227.0, 221.0, 215.0, 209.0, 204.0, 198.0, 192.0, 187.0, 181.0, 175.0, 170.0, 164.0, 158.0, 153.0, 147.0, 141.0, 136.0, 130.0, 124.0, 119.0, 113.0, 108.0, 102.0, 96.0, 91.0, 85.0, 79.0, 74.0, 68.0, 62.0, 57.0, 51.0, 45.0, 39.0, 34.0, 28.0, 22.0, 16.0, 11.0, 5.0, 0.0, -6.0, -11.0, -17.0, -22.0, -28.0, -33.0, -39.0, -44.0, -50.0, -55.0, -61.0, -66.0, -72.0, -77.0, -83.0, -88.0, -94.0, -99.0, -105.0, -110.0, -116.0, -121.0, -127.0, -132.0, -137.0, -143.0, -148.0, -154.0, -159.0, -165.0, -170.0, -176.0, -181.0, -186.0, -192.0, -197.0, -203.0, -208.0, -214.0, -219.0, -224.0, -230.0, -235.0, -241.0, -246.0, -251.0, -257.0, -262.0, -268.0, -273.0, -278.0, -284.0, -289.0, -295.0, -300.0, -305.0, -311.0, -316.0, -321.0, -327.0, -332.0, -337.0, -343.0, -348.0, -354.0, -359.0, -364.0, -370.0, -375.0, -380.0, -386.0, -391.0, -397.0, -402.0, -407.0, -413.0, -418.0, -423.0, -429.0, -434.0, -439.0, -445.0, -450.0, -455.0, -461.0, -466.0, -471.0, -477.0, -482.0, -487.0, -493.0, -498.0, -503.0, -509.0, -514.0, -519.0, -525.0, -530.0, -535.0, -540.0, -546.0, -551.0, -556.0, -562.0, -567.0, -572.0, -578.0, -583.0, -588.0, -593.0, -599.0, -604.0, -609.0, -615.0, -620.0, -625.0, -630.0, -636.0, -641.0, -646.0, -651.0, -657.0, -662.0, -667.0, -673.0, -678.0, -683.0, -688.0, -694.0, -699.0, -704.0, -709.0, -715.0, -720.0, -725.0, -730.0, -736.0, -741.0, -746.0, -751.0, -757.0, -762.0, -767.0, -772.0, -778.0, -783.0, -788.0, -793.0, -799.0, -804.0, -809.0, -814.0, -820.0, -825.0, -830.0, -835.0, -841.0, -846.0, -851.0, -856.0, -862.0, -867.0, -872.0, -877.0, -883.0, -888.0, -893.0, -898.0, -903.0, -909.0, -914.0, -919.0, -924.0, -930.0, -935.0, -940.0, -945.0, -951.0, -956.0, -961.0, -966.0, -971.0, -977.0, -982.0, -987.0, -992.0, -998.0, -1003.0, -1008.0, -1013.0, -1018.0, -1024.0, -1029.0, -1034.0, -1039.0, -1045.0, -1050.0, -1055.0, -1060.0, -1065.0, -1071.0, -1076.0, -1081.0, -1086.0, -1092.0, -1097.0, -1102.0, -1107.0, -1112.0, -1118.0, -1123.0, -1128.0, -1133.0, -1138.0, -1144.0, -1149.0, -1154.0, -1159.0, -1165.0, -1170.0, -1175.0, -1180.0, -1185.0, -1191.0, -1196.0, -1201.0, -1206.0, -1211.0, -1217.0, -1222.0, -1227.0, -1232.0, -1237.0, -1243.0, -1248.0, -1253.0, -1258.0, -1263.0, -1269.0, -1274.0, -1279.0, -1284.0, -1289.0, -1295.0, -1300.0, -1305.0, -1310.0, -1315.0, -1321.0, -1326.0, -1331.0, -1336.0, -1341.0, -1347.0, -1352.0, -1357.0, -1362.0, -1367.0, -1373.0, -1378.0, -1383.0, -1388.0, -1393.0, -1399.0, -1404.0, -1409.0, -1414.0, -1419.0, -1425.0, -1430.0, -1435.0, -1440.0, -1445.0, -1450.0, -1456.0, -1461.0, -1466.0, -1471.0, -1476.0, -1482.0, -1487.0, -1492.0, -1497.0, -1502.0, -1508.0, -1513.0, -1518.0, -1523.0, -1528.0, -1534.0, -1539.0, -1544.0, -1549.0, -1554.0, -1560.0, -1565.0, -1570.0, -1575.0, -1580.0, -1586.0, -1591.0, -1596.0, -1601.0, -1606.0, -1612.0, -1617.0, -1622.0, -1627.0, -1632.0, -1637.0, -1643.0, -1648.0, -1653.0, -1658.0, -1663.0, -1669.0, -1674.0, -1679.0, -1684.0, -1689.0, -1695.0, -1700.0, -1705.0, -1710.0, -1715.0, -1721.0, -1726.0, -1731.0, -1736.0, -1741.0, -1747.0, -1752.0, -1757.0, -1762.0, -1767.0, -1773.0, -1778.0, -1783.0, -1788.0, -1793.0, -1799.0, -1804.0, -1809.0, -1814.0, -1819.0, -1825.0, -1830.0, -1835.0, -1840.0, -1845.0, -1851.0, -1856.0, -1861.0, -1866.0, -1871.0, -1876.0, -1882.0, -1887.0, -1892.0, -1897.0, -1902.0, -1908.0, -1913.0, -1918.0, -1923.0, -1928.0, -1934.0, -1939.0, -1944.0, -1949.0, -1954.0, -1960.0, -1965.0, -1970.0, -1975.0, -1980.0, -1986.0, -1991.0, -1996.0, -2001.0, -2006.0, -2012.0, -2017.0, -2022.0, -2027.0, -2032.0, -2038.0, -2043.0, -2048.0, -2047.0, -2037.0, -2027.0, -2017.0, -2007.0, -1997.0, -1987.0, -1977.0, -1967.0, -1957.0, -1947.0, -1937.0, -1927.0, -1917.0, -1907.0, -1897.0, -1888.0, -1878.0, -1868.0, -1858.0, -1848.0, -1838.0, -1828.0, -1819.0, -1809.0, -1799.0, -1789.0, -1780.0, -1770.0, -1760.0, -1750.0, -1741.0, -1731.0, -1721.0, -1712.0, -1702.0, -1692.0, -1683.0, -1673.0, -1663.0, -1654.0, -1644.0, -1635.0, -1625.0, -1615.0, -1606.0, -1596.0, -1587.0, -1577.0, -1568.0, -1558.0, -1549.0, -1539.0, -1530.0, -1520.0, -1511.0, -1501.0, -1492.0, -1483.0, -1473.0, -1464.0, -1454.0, -1445.0, -1436.0, -1426.0, -1417.0, -1408.0, -1398.0, -1389.0, -1380.0, -1371.0, -1361.0, -1352.0, -1343.0, -1334.0, -1324.0, -1315.0, -1306.0, -1297.0, -1288.0, -1278.0, -1269.0, -1260.0, -1251.0, -1242.0, -1233.0, -1224.0, -1215.0, -1205.0, -1196.0, -1187.0, -1178.0, -1169.0, -1160.0, -1151.0, -1142.0, -1133.0, -1124.0, -1115.0, -1106.0, -1097.0, -1088.0, -1080.0, -1071.0, -1062.0, -1053.0, -1044.0, -1035.0, -1026.0, -1017.0, -1009.0, -1000.0, -991.0, -982.0, -973.0, -965.0, -953.0, -944.0, -935.0, -920.0, -906.0, -889.0, -871.0, -854.0, -842.0, -834.0, -826.0, -818.0, -810.0, -802.0, -794.0, -786.0, -778.0, -770.0, -762.0, -754.0, -746.0, -739.0, -731.0, -723.0, -715.0, -707.0, -699.0, -690.0, -682.0, -672.0, -661.0, -651.0, -639.0, -627.0, -616.0, -606.0, -598.0, -591.0, -584.0, -577.0, -570.0, -563.0, -556.0, -549.0, -542.0, -535.0, -528.0, -520.0, -513.0, -506.0, -499.0, -492.0, -485.0, -478.0, -471.0, -464.0, -457.0, -451.0, -444.0, -437.0, -430.0, -423.0, -416.0, -409.0, -400.0, -390.0, -382.0, -373.0, -364.0, -356.0, -349.0, -343.0, -336.0, -330.0, -323.0, -317.0, -310.0, -304.0, -297.0, -291.0, -284.0, -278.0, -271.0, -265.0, -258.0, -252.0, -245.0, -239.0, -232.0, -226.0, -219.0, -213.0, -207.0, -200.0, -194.0, -187.0, -181.0, -175.0, -168.0, -162.0, -156.0, -149.0, -143.0, -136.0, -128.0, -121.0, -114.0, -107.0, -100.0, -93.0, -87.0, -80.0, -74.0, -68.0, -62.0, -56.0, -50.0, -44.0, -38.0, -32.0, -26.0, -20.0, -14.0, -8.0, -2.0, 5.0, 11.0, 17.0, 23.0, 29.0, 35.0, 41.0, 47.0, 53.0, 59.0, 65.0, 70.0, 76.0, 82.0, 88.0, 94.0, 100.0, 106.0, 112.0, 118.0, 124.0, 130.0, 136.0, 142.0, 148.0, 154.0, 161.0, 167.0, 174.0, 180.0, 186.0, 192.0, 198.0, 204.0, 210.0, 215.0, 221.0, 227.0, 233.0, 238.0, 244.0, 250.0, 255.0, 261.0, 267.0, 273.0, 278.0, 284.0, 290.0, 295.0, 301.0, 307.0, 312.0, 318.0, 324.0, 329.0, 335.0, 341.0, 346.0, 352.0, 358.0, 363.0, 369.0, 374.0, 380.0, 386.0, 391.0, 397.0, 402.0, 408.0, 414.0, 419.0, 425.0, 430.0, 436.0, 441.0, 447.0, 453.0, 458.0, 464.0, 470.0, 475.0, 481.0, 487.0, 493.0, 499.0, 504.0, 510.0, 516.0, 521.0, 527.0, 532.0, 538.0, 543.0, 549.0, 554.0, 560.0, 565.0, 571.0, 576.0, 582.0, 587.0, 593.0, 598.0, 604.0, 609.0, 614.0, 620.0, 625.0, 631.0, 636.0, 642.0, 647.0, 653.0, 658.0, 663.0, 669.0, 674.0, 680.0, 685.0, 691.0, 696.0, 701.0, 707.0, 712.0, 718.0, 723.0, 728.0, 734.0, 739.0, 745.0, 750.0, 755.0, 761.0, 766.0, 772.0, 777.0, 782.0, 788.0, 793.0, 798.0, 804.0, 809.0, 815.0, 820.0, 826.0, 831.0, 837.0, 842.0, 847.0, 853.0, 858.0, 863.0, 869.0, 874.0, 880.0, 885.0, 890.0, 895.0, 901.0, 906.0, 911.0, 917.0, 922.0, 927.0, 933.0, 938.0, 943.0, 948.0, 954.0, 959.0, 964.0, 970.0, 975.0, 980.0, 985.0, 991.0, 996.0, 1001.0, 1006.0, 1012.0, 1017.0, 1022.0, 1027.0, 1033.0, 1038.0, 1043.0, 1048.0, 1054.0, 1059.0, 1064.0, 1069.0, 1075.0, 1080.0, 1085.0, 1090.0, 1096.0, 1101.0, 1106.0, 1111.0, 1116.0, 1122.0, 1127.0, 1132.0, 1137.0, 1143.0, 1148.0, 1153.0, 1158.0, 1163.0, 1169.0, 1174.0, 1179.0, 1184.0, 1190.0, 1195.0, 1200.0, 1205.0, 1211.0, 1216.0, 1221.0, 1226.0, 1231.0, 1237.0, 1242.0, 1247.0, 1252.0, 1257.0, 1262.0, 1268.0, 1273.0, 1278.0, 1283.0, 1288.0, 1293.0, 1298.0, 1304.0, 1309.0, 1314.0, 1319.0, 1324.0, 1329.0, 1334.0, 1340.0, 1345.0, 1350.0, 1355.0, 1360.0, 1365.0, 1370.0, 1375.0, 1381.0, 1386.0, 1391.0, 1396.0, 1401.0, 1406.0, 1411.0, 1416.0, 1421.0, 1427.0, 1432.0, 1437.0, 1442.0, 1447.0, 1452.0, 1457.0, 1462.0, 1467.0, 1472.0, 1478.0, 1483.0, 1488.0, 1493.0, 1498.0, 1503.0, 1508.0, 1513.0, 1518.0, 1523.0, 1528.0, 1534.0, 1539.0, 1544.0, 1549.0, 1554.0, 1559.0, 1564.0, 1569.0, 1574.0, 1579.0, 1584.0, 1589.0, 1595.0, 1600.0, 1605.0, 1610.0, 1615.0, 1620.0, 1625.0, 1630.0, 1635.0, 1640.0, 1645.0, 1650.0, 1655.0, 1660.0, 1666.0, 1671.0, 1676.0, 1681.0, 1686.0, 1691.0, 1696.0, 1701.0, 1706.0, 1711.0, 1716.0, 1721.0, 1726.0, 1731.0, 1736.0, 1741.0, 1746.0, 1751.0, 1757.0, 1762.0, 1767.0, 1772.0, 1777.0, 1782.0, 1787.0, 1792.0, 1797.0, 1802.0, 1807.0, 1812.0, 1817.0, 1822.0, 1827.0, 1832.0, 1837.0, 1842.0, 1847.0, 1852.0, 1857.0, 1862.0, 1867.0, 1872.0, 1877.0, 1883.0, 1888.0, 1893.0, 1898.0, 1903.0, 1908.0, 1913.0, 1918.0, 1923.0, 1928.0, 1933.0, 1938.0, 1943.0, 1948.0, 1953.0, 1958.0, 1963.0, 1968.0, 1973.0, 1978.0, 1983.0, 1988.0, 1993.0, 1998.0, 2003.0, 2008.0, 2013.0, 2018.0, 2023.0, 2028.0, 2033.0, 2038.0, 2043.0, 2048.0] ("appended array")
      # "smooth"
      # "24-09"
      # "Amp noise"
      n2 = xnode "Open FPGA VI Reference"() -> ("FPGA VI Reference Out"=w87:refnum<k20>, "error out"=w86:errorcluster)  [unwired: 2 in]
    }
  }
  n3 = xnode "Invoke Method"("FPGA VI Reference In"=w50, "error in"=w49) -> ("FPGA VI Reference Out"=w47:refnum<k20>, "error out"=w48:errorcluster)
  n4 = case shown="True" "Tri Low pass filter" {
    tunnel: w23 -> [w88 w93]
    tunnel: [w88 w89] -> w22
    tunnel: w21 -> [_ w94]
    frame False {
    }
    frame True {
      w90 = 1250 ("length")
      n5 = Build Array (concatenate)(w93, w93) -> (w92:dbl[])
      n6 = call-poly <vilib>:"Butterworth Filter.vi"("init/cont (init:F)"=FALSE, "filter type"=Filter_Passband_Type."Lowpass", "low cutoff freq: fl"="Low cutoff freq", "sampling freq: fs"=w94, "X"=w92) -> ("Filtered X"=w91:dbl[])  [unwired: 3 in, 1 out]
      n7 = Array Subset(array=w91, index=w90, length=w90) -> (w89:dbl[])
    }
  }
  n8 = xnode "Read/Write Control"("FPGA VI Reference In"=w47, "error in"=w48, "n"="#Signals") -> ("FPGA VI Reference Out"=w5:refnum<k20>, "error out"=w2:errorcluster)
  n9 = xnode "Read/Write Control"("FPGA VI Reference In"=w5, "error in"=w2, "n-bit (2^nbit medie)"="n-bit (2^nbit medie)") -> ("FPGA VI Reference Out"=w4:refnum<k20>, "error out"=w3:errorcluster)
  n10 = Add(x="lower limit 1", y=w75) -> (x+y=w79:u32)
  n11 = Add(x="lower limit 2", y=w75) -> (x+y=w77:u32)
  n12 = xnode "Read/Write Control"("FPGA VI Reference In"=w4, "error in"=w3, "upper limit 1"=w79, "upper limit 2"=w77, "lower limit 1"="lower limit 1", "lower limit 2"="lower limit 2", "Latency points"="Initial Latency points") -> ("FPGA VI Reference Out"=w74:refnum<k20>, "error out"=w73:errorcluster)
  n13 = xnode "Invoke Method"("FPGA VI Reference In"=w74, "error in"=w73, "Requested Depth"=u32 1000000) -> ("FPGA VI Reference Out"=w61:refnum<k20>, "error out"=w62:errorcluster)  [unwired: 1 out]
  n14 = xnode "Invoke Method"("FPGA VI Reference In"=w61, "error in"=w62, "Requested Depth"=u32 1000000) -> ("FPGA VI Reference Out"=w68:refnum<k20>, "error out"=w69:errorcluster)  [unwired: 1 out]
  n15 = xnode "Invoke Method"("FPGA VI Reference In"=w68, "error in"=w69) -> ("FPGA VI Reference Out"=w59:refnum<k20>, "error out"=w60:errorcluster)
  n16 = local read "Triangolo dritto?"() -> (w24:bool)
  n17 = xnode "Invoke Method"("FPGA VI Reference In"=w59, "error in"=w60) -> ("FPGA VI Reference Out"=w54:refnum<k20>, "error out"=w67:errorcluster)
  n18 = case shown="False" w24 {
    tunnel: [w100 dbl[] [1.0, 1.0, 1.0, 1.0, 1.0] ("mean factor 1")] -> w29
    tunnel: [w99 dbl[] [1.0, 1.0, 1.0, 1.0, 1.0] ("mean factor 1")] -> w28
    frame False {
      n19 = local read "Sample /Modulation Frequency"() -> (w98:enum32{"40MHz/32KHz", "30MHz/24Khz"})
      n20 = case shown="\"30MHz/24Khz\"" w98 {
        tunnel: [dbl[] [1.0, 0.7688144425878637, 0.960709657195022, 0.8322860112544478, 0.9000054001812109] ("mean factor 1") dbl[] [1.0, 0.7788051374952276, 0.9586568902543302, 0.8395566206470091, 0.903068410955916] ("mean factor 1")] -> w100
        tunnel: [dbl[] [0.9634618859268163, 0.8014672128927146, 0.9212223217673626, 0.8422741314179902, 0.8798034158007506] ("mean factor 2") dbl[] [1.0550150413710893, 0.8807744280543515, 1.0096480344577006, 0.9233799836458207, 0.9653106595082892] ("mean factor 2")] -> w99
        frame "40MHz/32KHz", Default {
          # "40M: Hanning"
        }
        frame "30MHz/24Khz" {
          (unwired) dbl[] [1.1005137000488208, 0.9187587728292271, 1.053190192155029, 0.9632017388419849, 1.0069407202113718] ("x/y 2")
          (unwired) dbl[] [1.043126075831679, 0.812391946912948, 1.0, 0.8757634031340201, 0.9420142077279946] ("x/y")
          # "rispetto il 3 tri"
          # "24-09"
        }
      }
    }
    frame True {
    }
  }
  n21 = xnode "Invoke Method"("FPGA VI Reference In"=w54, "error in"=w67) -> ("FPGA VI Reference Out"=w55:refnum<k20>, "error out"=w58:errorcluster)  [unwired: 1 in]
  n22 = To Long Integer(number="#Signals") -> (32bit integer=w43:i32)
  n23 = Multiply(x="#Signals", y=u32 1024 ("elements in array (1)")) -> (x*y=w39:u32)
  n24 = call "N-Wave Memory write from DMA - Host.vi"("Triangular Multiply Factor"="Triangular Multiply Factor", "Enable triangular scaling"="Enable triangular scaling", "n"=w43, "error in"=w58, "Custom Triangular Signal (fal-ris)"=w22, "Triangolo dritto?"="Triangolo dritto?", "FPGA VI Reference In"=w54) -> ("FPGA VI Reference Out"=w56:refnum<k20>, "error out"=w57:errorcluster)  [unwired: 2 in, 1 out]
  n25 = RT FIFO Create(1:dbl[] [] ("double precision float"), 4:u32 1000 ("size (10)"), 6:w39) -> (8:w36:refnum<k33>, 11:w37:errorcluster)  [unwired: 5 in, 1 out]
  n26 = call "Window Memory write from DMA - Host.vi"("error in"=w57, "Enum"="Windowing", "FPGA VI Reference In"=w56) -> ("FPGA VI Reference Out"=w13:refnum<k20>, "error out"=w14:errorcluster)  [unwired: 5 in, 2 out]
  n27 = call "Estrazione fondo (N-memory) - Host.vi"("polynomial order"="Savitzy golay: polynomial order", "LowPass Filter: Low cutoff frequency"="LowPass Filter: Low cutoff frequency", "side points"="Savitzy golay: side points", "PolyFitting: Poly Grade"="PolyFitting: Poly Grade", "SubtractionType"="SubtractionType", "error in"=w14, "FPGA VI Reference In"=w13) -> ("Fondo Signal"=→"Fondo Signal":dbl[], "error out"=w12:errorcluster)  [unwired: 1 in, 2 out]
  n28 = node-c288(i64 10 ("Period")) -> (w53:T6)  [unwired: 3 in]
  n29 = timed-loop {
    tunnel: w55 -> [w131]
    tunnel: w12 -> [w132]
    tunnel: [w134] -> w66
    tunnel: [w135] -> w65
    tunnel: [w120] -> w63
    tunnel: "#Signals" -> [w117]
    timing: w53 -> [_]
    timing-out: [_] -> w52
    shift-right: [w113] -> _
    shift-left: 0 -> [w116]
    tunnel: w36 -> [w112]
    tunnel: w37 -> [w109]
    tunnel: [w107] -> w31
    stop <- "stop" stop-if-true
    n30 = node-c288() -> ()  [unwired: 1 in, 1 out]
    n31 = flat-sequence {
      tunnel: w131 -> [w144]
      tunnel: w132 -> [w145]
      tunnel: "Snapshot" -> [w142]
      tunnel: "Snapshot" -> [w147]
      tunnel: [w146] -> w130
      tunnel: [w147] -> w129
      tunnel: [w142] -> w128
      tunnel: [w146] -> w127
      tunnel: [w143] -> w126
      tunnel: [w143] -> w125
      tunnel: [w141] -> w118
      tunnel: w117 -> [w141]
      tunnel: w116 -> [w140]
      tunnel: [w140] -> w115
      tunnel: w112 -> [w139]
      tunnel: [w139] -> w111
      tunnel: [w138] -> w110
      tunnel: w109 -> [w138]
      tunnel: w130 -> [w168]
      tunnel: w129 -> [w162]
      tunnel: w128 -> [w165]
      tunnel: w127 -> [w164]
      tunnel: w126 -> [w163]
      tunnel: w125 -> [w169]
      tunnel: [w167] -> w124
      tunnel: [w166] -> w123
      tunnel: [w161] -> w122
      tunnel: [w160] -> w119
      tunnel: w118 -> [w159]
      tunnel: w115 -> [w158]
      tunnel: [w158] -> w114
      tunnel: w111 -> [w157]
      tunnel: w110 -> [w156]
      tunnel: [w155] -> w108
      tunnel: [w257] -> w134
      tunnel: [w258] -> w135
      tunnel: w124 -> [w258]
      tunnel: w123 -> [w257]
      tunnel: w122 -> [w255]
      tunnel: [w256] -> w120
      tunnel: w119 -> [w256]
      tunnel: w114 -> [w254]
      tunnel: [w253] -> w113
      tunnel: w108 -> [w252]
      tunnel: [w252] -> w107
      frame #0 {
        n32 = case shown="False" w142 {
          tunnel: [w148 w154] -> w146
          tunnel: w145 -> [w148 w153]
          tunnel: w144 -> [w149 w152]
          tunnel: [w149 w151] -> w143
          frame False {
          }
          frame True {
            n33 = xnode "Read/Write Control"("FPGA VI Reference In"=w152, "error in"=w153, "snapshot"=TRUE) -> ("FPGA VI Reference Out"=w151:refnum<k20>, "error out"=w154:errorcluster)
          }
        }
      }
      frame #1 {
        n34 = flat-sequence {
          tunnel: w169 -> [w178]
          tunnel: w168 -> [w177]
          tunnel: w162 -> [w174]
          tunnel: [w176] -> w172
          tunnel: [w175] -> w171
          tunnel: [w174] -> w170
          tunnel: w159 -> [w173]
          tunnel: [w209] -> w166
          tunnel: w172 -> [w211]
          tunnel: w171 -> [w210]
          tunnel: w170 -> [w208]
          tunnel: [w208] -> w161
          tunnel: [w207] -> w160
          frame #0 {
            n35 = case shown="True" w174 {
              tunnel: w178 -> [w182 w206]
              tunnel: w177 -> [w181 w205]
              tunnel: [w180 w204] -> w175
              tunnel: [w179 w203] -> w176
              tunnel: w173 -> [_ w202]
              frame False {
                n36 = disable-structure shown="Enabled" {
                  disable-tunnel: w182 -> [w189 w192]
                  disable-tunnel: w181 -> [w187 w191]
                  disable-tunnel: [w186 w191] -> w180
                  disable-tunnel: [w183 w192] -> w179
                  frame Disabled {
                    n37 = xnode "Invoke Method"("FPGA VI Reference In"=w189, "error in"=w187, "Number of Elements"=u32 0) -> ("FPGA VI Reference Out"=w185:refnum<k20>, "error out"=w184:errorcluster, "Elements Remaining"=w188:u32)  [unwired: 1 in, 1 out]
                    n38 = xnode "Invoke Method"("FPGA VI Reference In"=w185, "error in"=w184, "Number of Elements"=w188) -> ("FPGA VI Reference Out"=w183:refnum<k20>, "error out"=w186:errorcluster)  [unwired: 1 in, 2 out]
                  }
                  frame Enabled {
                  }
                }
              }
              frame True {
                n39 = Multiply(x=w202, y=u32 1024 ("Number of Elements")) -> (x*y=w196:u32)
                n40 = xnode "Invoke Method"("FPGA VI Reference In"=w206, "error in"=w205, "Number of Elements"=w196, "Timeout (ms)"=-1) -> ("FPGA VI Reference Out"=w199:refnum<k20>, "error out"=w198:errorcluster, "Data"=w201:fxp<+/-,12,12>[])  [unwired: 1 out]
                n41 = To Double Precision Float(number=w201) -> (double precision float=→"N-Signals":dbl[])
                n42 = xnode "Invoke Method"("FPGA VI Reference In"=w199, "error in"=w198, "Number of Elements"=u32 0) -> ("FPGA VI Reference Out"=w203:refnum<k20>, "error out"=w204:errorcluster, "Elements Remaining"=→"Elements Remaining Signal":u32)  [unwired: 1 in, 1 out]
              }
            }
          }
          frame #1 {
            n43 = case shown="False" w208 {
              tunnel: [w213 w216] -> w209
              tunnel: w211 -> [w212 w217]
              tunnel: w210 -> [w213 w215]
              tunnel: [w212 w214] -> w207
              frame False {
              }
              frame True {
                n44 = xnode "Read/Write Control"("FPGA VI Reference In"=w217, "error in"=w215, "snapshot"=FALSE) -> ("FPGA VI Reference Out"=w214:refnum<k20>, "error out"=w216:errorcluster)
              }
            }
          }
        }
        n45 = case shown="True" w165 {
          tunnel: w163 -> [w222 w250]
          tunnel: w164 -> [w221 w251]
          tunnel: [w220 w249] -> w167
          tunnel: w159 -> [_ w237]
          tunnel: w157 -> [w219 w235]
          tunnel: w156 -> [_ w234]
          tunnel: [w219 w232] -> w155
          frame False {
            n46 = disable-structure shown="Enabled" {
              disable-tunnel: w222 -> [w228 _]
              disable-tunnel: w221 -> [w225 w230]
              disable-tunnel: [w224 w230] -> w220
              frame Disabled {
                n47 = xnode "Invoke Method"("FPGA VI Reference In"=w228, "error in"=w225, "Number of Elements"=u32 0) -> ("FPGA VI Reference Out"=w226:refnum<k20>, "error out"=w223:errorcluster, "Elements Remaining"=w227:u32)  [unwired: 1 in, 1 out]
                n48 = xnode "Invoke Method"("FPGA VI Reference In"=w226, "error in"=w223, "Number of Elements"=w227) -> ("error out"=w224:errorcluster)  [unwired: 1 in, 3 out]
              }
              frame Enabled {
              }
            }
          }
          frame True {
            # "256x5"
            # "256x5"
            n49 = Multiply(x=w237, y=u32 1024 ("Number of Elements")) -> (x*y=w241:u32)
            n50 = xnode "Invoke Method"("FPGA VI Reference In"=w250, "error in"=w251, "Number of Elements"=w241, "Timeout (ms)"=-1) -> ("FPGA VI Reference Out"=w245:refnum<k20>, "error out"=w246:errorcluster, "Data"=w248:fxp<+,44,44>[])  [unwired: 1 out]
            n51 = To Double Precision Float(number=w248) -> (double precision float=w247:dbl[])
            n52 = Square Root(x=w247) -> (sqrt(x)=w238:dbl[])
            n53 = xnode "Invoke Method"("FPGA VI Reference In"=w245, "error in"=w246, "Number of Elements"=u32 0) -> ("error out"=w249:errorcluster, "Elements Remaining"=→"Elements Remaining FFT":u32)  [unwired: 1 in, 2 out]
            n54 = call "CleanCompleteFFTArray.vi"("Complete FFT Array"=w238, "FFT Size"=512, "#Signals"=w237) -> ("Second Edge Array"=w236:dbl[], "First Edge Array"=w231:dbl[])  [unwired: 7 in]
            "FALLING First Edge N-FFT" <- w231
            "RISING Second Edge N-FFT" <- w236
            n55 = Build Array (concatenate)(w231, w236) -> (w233:dbl[])
            n56 = RT FIFO Write(0:w235, 1:w233, 3:w234) -> (8:w232:refnum<k33>)  [unwired: 2 in, 3 out]
          }
        }
      }
      frame #2 {
        n57 = case shown="False" w255 {
          tunnel: w254 -> [w259 w263]
          tunnel: [w259 w264] -> w253
          frame False {
          }
          frame True {
            n58 = Decrement(x="tieni premuto per") -> (x-1=w260:i32)
            n59 = Greater Or Equal?(x=w263, y=w260) -> (x >= y?=w262:bool)
            n60 = case shown="True" w262 {
              tunnel: w263 -> [w265 _]
              tunnel: [w266 0] -> w264
              frame False {
                n61 = Increment(x=w265) -> (x+1=w266:i32)
              }
              frame True {
                n62 = local write "Snapshot"(FALSE ("Snapshot")) -> ()
              }
            }
          }
        }
      }
    }
    n63 = node-c288() -> ()  [unwired: 1 in, 1 out]
  }
  n64 = while {
    tunnel: w36 -> [w296]
    tunnel: "first bin" -> [w293]
    tunnel: "last bin" -> [w292]
    tunnel: "Windowing" -> [w291]
    tunnel: "#Signals" -> [w290]
    shift-right: [w288] -> _
    shift-left: w25 -> [w275]
    tunnel: w21 -> [w287]
    tunnel: w29 -> [w286]
    tunnel: w28 -> [w285]
    shift-right: [w283] -> _
    shift-left: 0 ("first bin") -> [w284]
    tunnel: w26 -> [w282]
    shift-right: [w281] -> _
    shift-left: w25 -> [w274]
    shift-right: [w269] -> w18
    shift-left: dbl[] [] -> [w270]
    stop <- w289 stop-if-true
    # "VelocityMoving average"
    # "Distance Moving average"
    n65 = Wait (ms)(milliseconds to wait=u32 10 ("millisecond multiple")) -> ()  [unwired: 1 out]
    n66 = RT FIFO Read(0:w296) -> (9:w294:dbl[], 10:w295:bool)  [unwired: 3 in, 3 out]
    n67 = Array Size(array=w274) -> (size(s)=w280:i32)
    n68 = Array Size(array=w275) -> (size(s)=w276:i32)
    "mean distance size" <- w276
    n69 = Greater Or Equal?(x=w280, y="#movesignal 2") -> (x >= y?=w279:bool)
    n70 = Greater Or Equal?(x=w276, y="#movesignal") -> (x >= y?=w277:bool)
    n71 = case shown="True" w279 {
      tunnel: w274 -> [w298 w306]
      tunnel: [w298 w303] -> w272
      frame False {
      }
      frame True {
        n72 = call <vilib>:"Std Deviation and Variance.vi"("X"=w306) -> ("mean"=w299:dbl, "standard deviation"=w301:dbl)  [unwired: 1 in, 1 out]
        "moving mean speed" <- w299
        n73 = Subtract(x=w299, y=w301) -> ()  [unwired: 1 out]
        n74 = Add(x=w299, y=w301) -> ()  [unwired: 1 out]
        n75 = Absolute Value(x=w299) -> (abs(x)=w308:dbl)
        n76 = Build Array(w299) -> (w302:dbl[])
        n77 = Divide(x=w301, y=w308) -> (x/y=→"moving standard deviation rel speed":dbl)
        n78 = Array To Cluster(array=w302) -> (cluster=→"Speed and error":T2)
        n79 = Delete From Array(array=w306, length=1, index=0) -> (array with subset deleted=w303:dbl[])  [unwired: 1 out]
      }
    }
    n80 = case shown="True" w277 {
      tunnel: w275 -> [w310 w316]
      tunnel: [w310 w323] -> w273
      tunnel: w270 -> [w309 w315]
      tunnel: [w309 w313] -> w269
      frame False {
      }
      frame True {
        # "coeff empirico"
        n81 = call <vilib>:"Std Deviation and Variance.vi"("X"=w316) -> ("mean"=w314:dbl, "standard deviation"=w318:dbl)  [unwired: 1 in, 1 out]
        "moving mean" <- w314
        n82 = Absolute Value(x=w314) -> (abs(x)=w325:dbl)
        n83 = Divide(x=w318, y=w325) -> (x/y=→"moving standard deviation rel":dbl)
        n84 = Divide(x=w314, y=2.614797e-07 ("Empirical Distance Costant")) -> (x/y=→"moving freq mean":dbl)
        n85 = case shown="True" "Lin Mes" {
          tunnel: w315 -> [w327 w330]
          tunnel: w314 -> [_ w329]
          tunnel: [w327 w328] -> w313
          frame False {
          }
          frame True {
            n86 = Build Array (concatenate)(w330, w329) -> (w328:dbl[])
          }
        }
        n87 = case shown="False" "Mov mean" {
          tunnel: w316 -> [_ w335]
          tunnel: [dbl[] [] ("appended array") w332] -> w323
          frame False {
            # "Mean"
          }
          frame True {
            # "Mov Mean"
            n88 = Delete From Array(array=w335, length=1, index=0) -> (array with subset deleted=w332:dbl[])  [unwired: 1 out]
          }
        }
        n89 = Build Array(w314, w318) -> (w322:dbl[])
        n90 = Array To Cluster(array=w322) -> (cluster=w321:T2)
        n91 = case shown="True" "Plot" {
          tunnel: w321 -> [_ w326]
          frame False {
          }
          frame True {
            "Distance and error" <- w326
          }
        }
        "Distance ONLINE" <- w316
      }
    }
    n92 = case shown="False" w295 {
      tunnel: w294 -> [w376 _]
      tunnel: w293 -> [w372 _]
      tunnel: w292 -> [w371 _]
      tunnel: w291 -> [w370 _]
      tunnel: w290 -> [w367 _]
      tunnel: [w359 w513] -> w288
      tunnel: w287 -> [w356 _]
      tunnel: w286 -> [w355 _]
      tunnel: w285 -> [w354 _]
      tunnel: w284 -> [w353 w514]
      tunnel: [w341 w514] -> w283
      tunnel: w282 -> [w340 _]
      tunnel: [w339 w512] -> w281
      tunnel: w273 -> [w338 w513]
      tunnel: w272 -> [w337 w512]
      frame False {
        w366 = dbl[] [] ("appended array")
        # "window"
        # "ris"
        # "fall"
        n93 = Array Size(array=w376) -> (size(s)=w374:i32)
        n94 = Divide(x=w374, y=2) -> (x/y=w375:dbl)
        n95 = Split 1D Array(array=w376, index=w375) -> (first subarray=w368:dbl[], second subarray=w369:dbl[])
        n96 = while {
          shift-right: [w444] -> _
          shift-left: w368 -> [w456]
          shift-right: [w445] -> _
          shift-left: w369 -> [w455]
          tunnel: w372 -> [w452]
          tunnel: w371 -> [w451]
          tunnel: w370 -> [w431]
          tunnel: w367 -> [w449]
          shift-right: [w430] -> w365
          shift-left: w366 -> [w428]
          shift-right: [w429] -> w364
          shift-left: w366 -> [w427]
          tunnel: w355 -> [w426] mode=indexing
          tunnel: w354 -> [w425] mode=indexing
          tunnel: [w424] -> w351 mode=indexing
          tunnel: [w423] -> w349 mode=indexing
          tunnel: w340 -> [w422]
          tunnel: [w420] -> w336 mode=indexing
          i -> [w446]
          stop <- w450 stop-if-true
          w448 = 256 ("x")
          # "ris"
          # "fall"
          # "max bin detect"
          # "Check amplitude & delta"
          # "Amplitude noise"
          n97 = Increment(x=w446) -> (x+1=w447:i32)
          n98 = Equal?(x=w447, y=w449) -> (x = y?=w450:bool)
          n99 = Split 1D Array(array=w456, index=w448) -> (first subarray=w454:dbl[], second subarray=w444:dbl[])
          n100 = Split 1D Array(array=w455, index=w448) -> (first subarray=w453:dbl[], second subarray=w445:dbl[])
          n101 = call "Max Bin Detection.vi"("FFT Array"=w454, "Init Discard Bins"=w452, "Last Discard Bins"=w451) -> ("Max Bin"=w420:i32, "Prev Max Amp"=w434:dbl, "Max Amp"=w433:dbl, "Succ Max Amp"=w432:dbl)  [unwired: 11 in, 2 out]
          n102 = call "Max Bin Detection.vi"("FFT Array"=w453, "Init Discard Bins"=w452, "Last Discard Bins"=w451) -> ("Max Bin"=w435:i32, "Prev Max Amp"=w438:dbl, "Max Amp"=w436:dbl, "Succ Max Amp"=w437:dbl)  [unwired: 11 in, 2 out]
          n103 = case shown="False" "3 point interpolation algorithm" {
            tunnel: [FALSE ("Check Delta Amp Ok?") w464] -> w440
            tunnel: [FALSE ("Check Delta Amp Ok?") w463] -> w439
            tunnel: w438 -> [_ w462]
            tunnel: w437 -> [_ w461]
            tunnel: w434 -> [_ w460]
            tunnel: w432 -> [_ w459]
            frame False {
            }
            frame True {
              w465 = 10.0 ("Max Difference %")
              # "delta diff%"
              n104 = call "Check Delta Amplitude Extreme bins.vi"("Succ Max Amp"=w459, "Max Difference %"=w465, "Prev Max Amp"=w460) -> ("Check Delta Amp Ok?"=w464:bool)  [unwired: 1 in, 1 out]
              n105 = call "Check Delta Amplitude Extreme bins.vi"("Succ Max Amp"=w461, "Max Difference %"=w465, "Prev Max Amp"=w462) -> ("Check Delta Amp Ok?"=w463:bool)  [unwired: 1 in, 1 out]
            }
          }
          n106 = call "Check Amplitude Bin.vi"("Threshold Amp"=w422, "Max Amp"=w433) -> ("Check Amp Ok?"=w443:bool)  [unwired: 2 in]
          n107 = call "Check Amplitude Bin.vi"("Threshold Amp"=w422, "Max Amp"=w436) -> ("Check Amp Ok?"=w442:bool)  [unwired: 2 in]
          n108 = And(x=w443, y=w442) -> (x .and. y?=w441:bool)
          n109 = case shown="True" w441 {
            tunnel: w440 -> [_ w489]
            tunnel: w439 -> [_ w488]
            tunnel: w438 -> [_ w487]
            tunnel: w437 -> [_ w486]
            tunnel: w436 -> [_ w485]
            tunnel: w435 -> [_ w484]
            tunnel: w420 -> [_ w483]
            tunnel: w434 -> [_ w482]
            tunnel: w433 -> [_ w481]
            tunnel: w432 -> [_ w480]
            tunnel: w431 -> [_ w479]
            tunnel: [w468 w474] -> w430
            tunnel: [w467 w473] -> w429
            tunnel: w428 -> [w468 w478]
            tunnel: w427 -> [w467 w477]
            tunnel: w426 -> [_ w476]
            tunnel: w425 -> [_ w475]
            tunnel: [w466 w470] -> w424
            tunnel: [w466 w469] -> w423
            frame False {
              w466 = 0.0
            }
            frame True {
              # "Bin correction"
              # "Interpolation"
              n110 = case shown="False" w489 {
                tunnel: w483 -> [w505 w511]
                tunnel: w482 -> [w503 w510]
                tunnel: w481 -> [w502 w509]
                tunnel: w480 -> [w501 w508]
                tunnel: [w504 w507] -> w472
                tunnel: w479 -> [w506 _]
                frame False {
                  n111 = call "IFFT Bin interpolation.vi"("Max Bin"=w505, "Max Amp"=w502, "Prev Max Amp"=w503, "Succ Max Amp"=w501, "Windowing"=w506) -> ("Interpolate Bin"=w504:dbl)
                }
                frame True {
                  n112 = call "Barycentric method RT.vi"("Next Amp"=w508, "Max Bin"=w511, "Max Amp"=w509, "Prev Amp"=w510) -> ("Bin"=w507:dbl)  [unwired: 7 in]
                }
              }
              n113 = case shown="False" w488 {
                tunnel: w487 -> [w491 w500]
                tunnel: w486 -> [w490 w499]
                tunnel: w485 -> [w492 w498]
                tunnel: w484 -> [w494 w497]
                tunnel: [w493 w496] -> w471
                tunnel: w479 -> [w495 _]
                frame False {
                  n114 = call "IFFT Bin interpolation.vi"("Max Bin"=w494, "Max Amp"=w492, "Prev Max Amp"=w491, "Succ Max Amp"=w490, "Windowing"=w495) -> ("Interpolate Bin"=w493:dbl)
                }
                frame True {
                  n115 = call "Barycentric method RT.vi"("Next Amp"=w499, "Max Bin"=w497, "Max Amp"=w498, "Prev Amp"=w500) -> ("Bin"=w496:dbl)  [unwired: 7 in]
                }
              }
              n116 = Divide(x=w472, y=w476) -> (x/y=w470:dbl)
              n117 = Divide(x=w471, y=w475) -> (x/y=w469:dbl)
              n118 = Build Array (concatenate)(w477, w469) -> (w473:dbl[])
              n119 = Build Array (concatenate)(w478, w470) -> (w474:dbl[])
            }
          }
        }
        "Array" <- w336
        n120 = Array Size(array=w365) -> (size(s)=w362:i32)
        "Fall array size" <- w362
        n121 = Array Size(array=w364) -> (size(s)=→"Rise array size":i32)
        n122 = Array To Cluster(array=w351) -> (cluster=→"5 bin FALL":T2)
        n123 = Array To Cluster(array=w349) -> (cluster=→"5 bin RISE":T2)
        n124 = Greater Than 0?(x=w362) -> (x > 0?=w360:bool)
        n125 = case shown="True" w360 {
          tunnel: w365 -> [_ w418]
          tunnel: w364 -> [_ w417]
          tunnel: w338 -> [w397 w405]
          tunnel: [w397 w404] -> w359
          tunnel: w356 -> [_ w403]
          tunnel: w337 -> [w396 w401]
          tunnel: [w396 w399] -> w339
          frame False {
          }
          frame True {
            w419 = 512.0 ("FFT size")
            # "coeff empirico"
            n126 = call <vilib>:"Std Deviation and Variance.vi"("X"=w418) -> ("mean"=w406:dbl, "standard deviation"=w407:dbl)  [unwired: 1 in, 1 out]
            n127 = call <vilib>:"Std Deviation and Variance.vi"("X"=w417) -> ("mean"=w411:dbl, "standard deviation"=w413:dbl)  [unwired: 1 in, 1 out]
            n128 = Absolute Value(x=w411) -> (abs(x)=w412:dbl)
            n129 = Absolute Value(x=w406) -> (abs(x)=w408:dbl)
            n130 = call "Frequency from bin number RT.vi"("FFT size"=w419, "Bin number"=w406, "Sample Rate (S/s)"=w403) -> ("Detected Frequency (Hz)"=w416:dbl)  [unwired: 8 in]
            "Mean Frequency Falling (Hz)" <- w416
            n131 = Divide(x=w413, y=w412) -> (x/y=→"StdDev Rel 2":dbl)
            n132 = call "Frequency from bin number RT.vi"("FFT size"=w419, "Bin number"=w411, "Sample Rate (S/s)"=w403) -> ("Detected Frequency (Hz)"=w415:dbl)  [unwired: 8 in]
            "Mean Frequency Rising (Hz)" <- w415
            n133 = Divide(x=w407, y=w408) -> (x/y=→"StdDev Rel 1":dbl)
            n134 = call "Distance-Velocity from Freq.vi"("freq_rising"=w415, "Empirical Distance Costant"=2.614797e-07, "freq_falling"=w416) -> ("Distance (m)"=w402:dbl, "Mean Frequency"=→"Mean Frequency":dbl, "Velocity (m/s)"=w400:dbl)  [unwired: 2 in]
            "Distance (m)" <- w402
            "Velocity (m/s)" <- w400
            n135 = Build Array (concatenate)(w401, w400) -> (w399:dbl[])
            n136 = Build Array (concatenate)(w405, w402) -> (w404:dbl[])
          }
        }
        n137 = Increment(x=w353) -> (x+1=w342:i32)
        n138 = Equal?(x=w342, y="#meanBin") -> (x = y?=w352:bool)
        n139 = Not(x=w360) -> (.not. x?=→"Warning":bool)
        n140 = feedback #1(T9 [] ("Real Matrix")) -> (w347:T9)
        n141 = feedback #2(T9 [] ("Real Matrix")) -> (w345:T9)
        n142 = case shown="True" w352 {
          tunnel: w349 -> [w382 _]
          tunnel: w351 -> [w383 _]
          tunnel: [w381 w395] -> w346
          tunnel: [w380 w395] -> w348
          tunnel: w347 -> [w379 w394]
          tunnel: w345 -> [w378 w393]
          tunnel: w342 -> [w377 _]
          tunnel: [w377 0] -> w341
          frame False {
            n143 = Build Array (concatenate)(w379, w383) -> (w380:T9)
            n144 = Build Array (concatenate)(w378, w382) -> (w381:T9)
          }
          frame True {
            w395 = T9 [] ("Real Matrix")
            n145 = call "MatrixMean.vi"("Real Matrix"=w394) -> ("DevStd Assoluta"=w385:dbl[], "Mean"=w384:dbl[])  [unwired: 8 in, 1 out]
            n146 = call "MatrixMean.vi"("Real Matrix"=w393) -> ("DevStd Assoluta"=w388:dbl[], "Mean"=w389:dbl[])  [unwired: 8 in, 1 out]
            n147 = Build Array (concatenate)(w384, w385) -> (w386:dbl[])
            n148 = Build Array (concatenate)(w389, w388) -> (w387:dbl[])
            n149 = Array To Cluster(array=w386) -> (cluster=→"5 bin mean/std FALL":T2)
            n150 = Array To Cluster(array=w387) -> (cluster=→"5 bin mean/std RISE":T2)
          }
        }
        n151 = feedback-in #1(w348) -> ()
        n152 = feedback-in #2(w346) -> ()
      }
      frame True {
      }
    }
    n153 = local read "stop"() -> (w289:bool)
  }
  n154 = node-c288(w52) -> ()  [unwired: 1 out]
  n155 = Merge Errors(w65, w66) -> (w70:errorcluster)
  n156 = flat-sequence {
    tunnel: w70 -> [w522]
    tunnel: w63 -> [w517]
    tunnel: w31 -> [w515]
    frame #0 {
      n157 = xnode "Invoke Method"("FPGA VI Reference In"=w517, "error in"=w522) -> ("FPGA VI Reference Out"=w519:refnum<k20>, "error out"=w518:errorcluster)
      n158 = RT FIFO Delete(0:w515) -> ()  [unwired: 2 in, 1 out]
      n159 = property on="stop" class="Bool (strict)"("Value"=FALSE ("stop")) -> ()  [unwired: 2 in, 2 out]
      n160 = xnode "Invoke Method"("FPGA VI Reference In"=w519, "error in"=w518) -> ("FPGA VI Reference Out"=w520:refnum<k20>, "error out"=w521:errorcluster)
      n161 = xnode "Close FPGA VI Reference"("FPGA VI Reference In"=w520, "error in"=w521) -> ()  [unwired: 1 out]
    }
  }
  n162 = call "Linearize Measure Evaluation.vi"("step (m)"="step (m)", "Distance Array"=w18) -> ("Mean error (m)"=→"Mean error (m)":dbl, "Max peak-peak error (m)"=→"Max peak-peak error (m)":dbl)  [unwired: 6 in, 2 out]
